vi "Demo Main BSC.vi"() -> ()   [LabVIEW 2022 SP3]
uses:
  Logo.ctl
  C:/Users/Public/OneDrive/Desktop/PMT program/SampleCodeLabView/Kinesis_with_LabVIEW_Examples_LV12 - v3/Thorlabs.MotionControl.Controls.dll
  Kinesis_with_LabVIEW_Examples_LV12 - v3/Thorlabs.MotionControl.Controls.dll
  C:/Users/Public/OneDrive/Desktop/PMT program/SampleCodeLabView/Kinesis_with_LabVIEW_Examples_LV12 - v3/Thorlabs.MotionControl.Benchtop.StepperMotorCLI.dll
  Kinesis_with_LabVIEW_Examples_LV12 - v3/Thorlabs.MotionControl.Benchtop.StepperMotorCLI.dll
  <vilib>/Utility/file.llb/Write Delimited Spreadsheet (string).vi
  <vilib>/Utility/file.llb/Write Delimited Spreadsheet (I64).vi
  <vilib>/Utility/file.llb/Write Delimited Spreadsheet (DBL).vi
  C:/Users/Public/OneDrive/Desktop/PMT program/SampleCodeLabView/Kinesis_with_LabVIEW_Examples_LV12 - v3/Thorlabs.MotionControl.GenericMotorCLI.dll
  Kinesis_with_LabVIEW_Examples_LV12 - v3/Thorlabs.MotionControl.GenericMotorCLI.dll
  <vilib>/Analysis/NI_AALBase.lvlib
panel:
  out "ESD":i32=1 caption="Steps\nAdded/Removed"
  in  "ES":i32=1 caption="Add /Remove \nSteps" format="%.0g"
  out "Sweep Graph":u32[](graph)=[692, 692, 717, 859, 1299, 1810, 1150, 733, 722, 683, 685, 676, 665, 671, 1299, 1362, 1395, 1437, 1460, 1539, 1625, 1626, 1658, 1682, 1737, 1780, 1784, 1780, 1793, 1801, 1778, 1738, 1746, 1700, 1643, 1578, 1545, 1504, 1448, 1394, 1310, 1272, 1209, 1133, 1067, 1028, 991, 955, 889, 855, 832, 810, 790, 767, 743, 738, 724, 715, 709, 699, 697, 691, 696, 694, 695, 710, 710, 694, 696, 690, 687, 684, 682, 689, 668]
  out "SM":i32 caption="Sweep\nMean"
  out "SN":i32=61 caption="Current Sweep Iteration"
  out "SND":i32=61 caption="Total No. of Sweeps"
  in  "Auto-Sweep":bool
  in  "P8":bool
  out "PC":dbl=1810482.0 caption="Current \nPosition" format="%#_6f"
  out "WTD":i32=2000 caption="Wait Time (ms)\nRead Data"
  out "EPD":dbl=70.72 caption="End Position\nRead Data"
  out "SPD":dbl=70.66 caption="Start Position\nRead Data"
  out "SSD":dbl=0.001 caption="Step Size\nRead Data" format="%.4g"
  in  "SP":dbl=70.66 caption="Start Position (degrees)\n Set Data"
  in  "WT":i32=2000 caption="Wait Time (ms)\n Set Data"
  in  "EP":dbl=70.72 caption="End Position (degrees)\n Set Data"
  in  "P7":bool
  in  "SS":dbl=0.001 caption="Step Size (degrees)\nSet Data"
  in  "Motor Controller\nSerialNumber":string="40837323"
  in  "BenchtopStepperControl":refnum<k24>(container)
  in  "Export":bool
  out "DB":u32[](array[numeric])=[729, 0, 0, 0, 0, 0, 0, 0, 0, 0, 0, 0, 0, 0, 0, 0]
  out "OVL":bool caption="LED ON : Over Rang Data"
  out "OLD":i32
  out "GN":i32 caption="Gate Number"
  in  "Correction":bool=TRUE
  in  "Logo":T1
  out "Graph":u32[](graph)=[729]
  in  "Stop":bool
  in  "Start":bool
  in  "P6":bool
  out "RND":i32=40 caption="Read Number\nRead Data"
  in  "P5":bool
  in  "RN":i32=40 caption="Read Number\nSet Data"
  out "PowerD":i32=1 caption="Power\nRead Data"
  out "ITD":i32=100 caption="Internal Time\nRead Data"
  in  "P4":bool
  in  "P3":bool
  in  "IT":i32=100 caption="Internal Time\nSet Data"
  in  "P2":bool
  out "Handle Number":i32=169470376
  in  "P1":bool caption="Switch\nPower OFF/Power ON"
  in  "EXIT":bool=TRUE
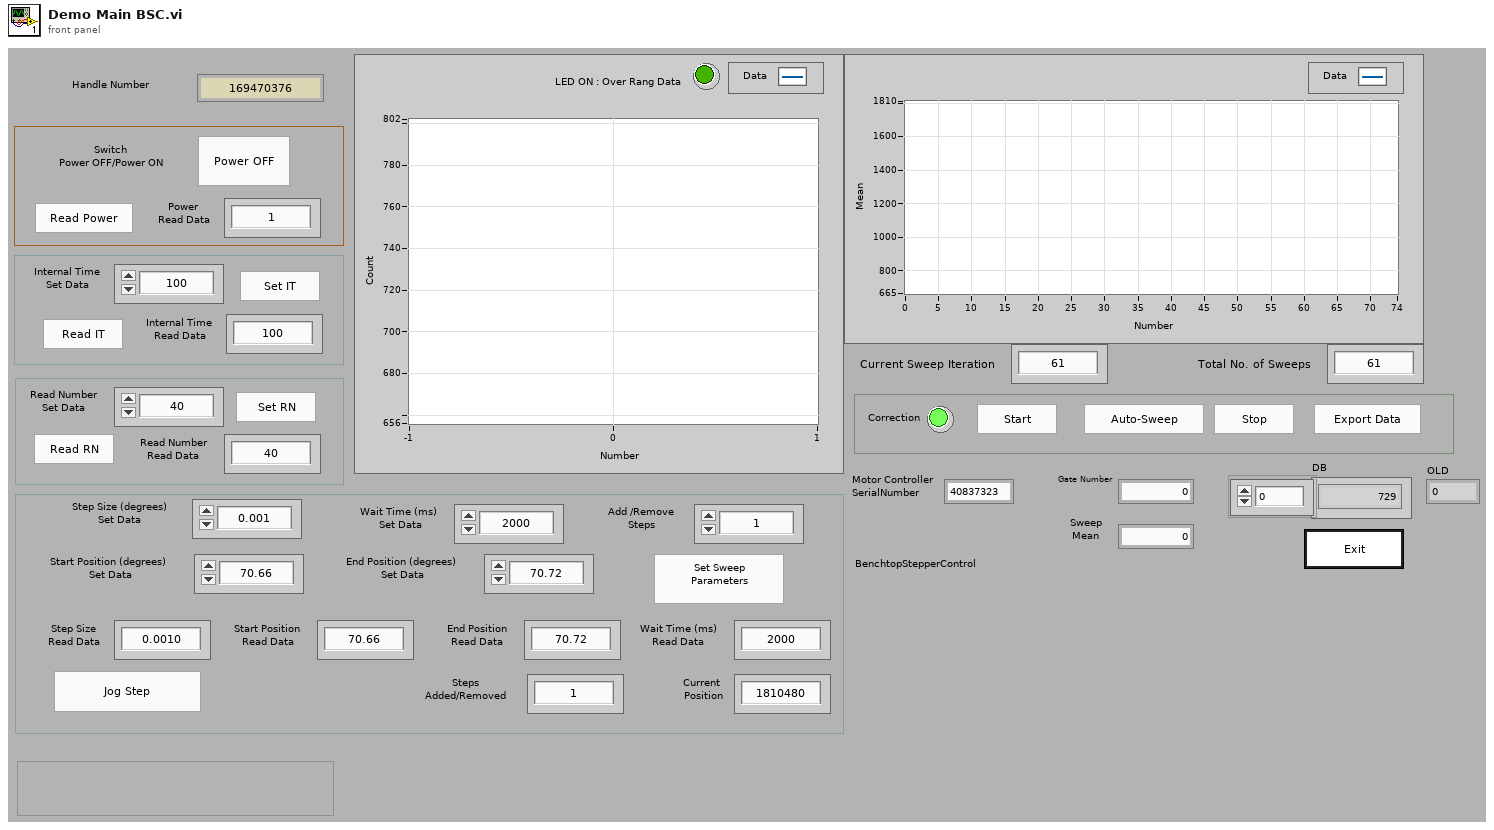
[diagram p1: front panel]
types:
  T1 = typedef "Logo.ctl" = bool
  T2 = enum8{"Enabled", "Disabled", "Disabled and Grayed Out"}
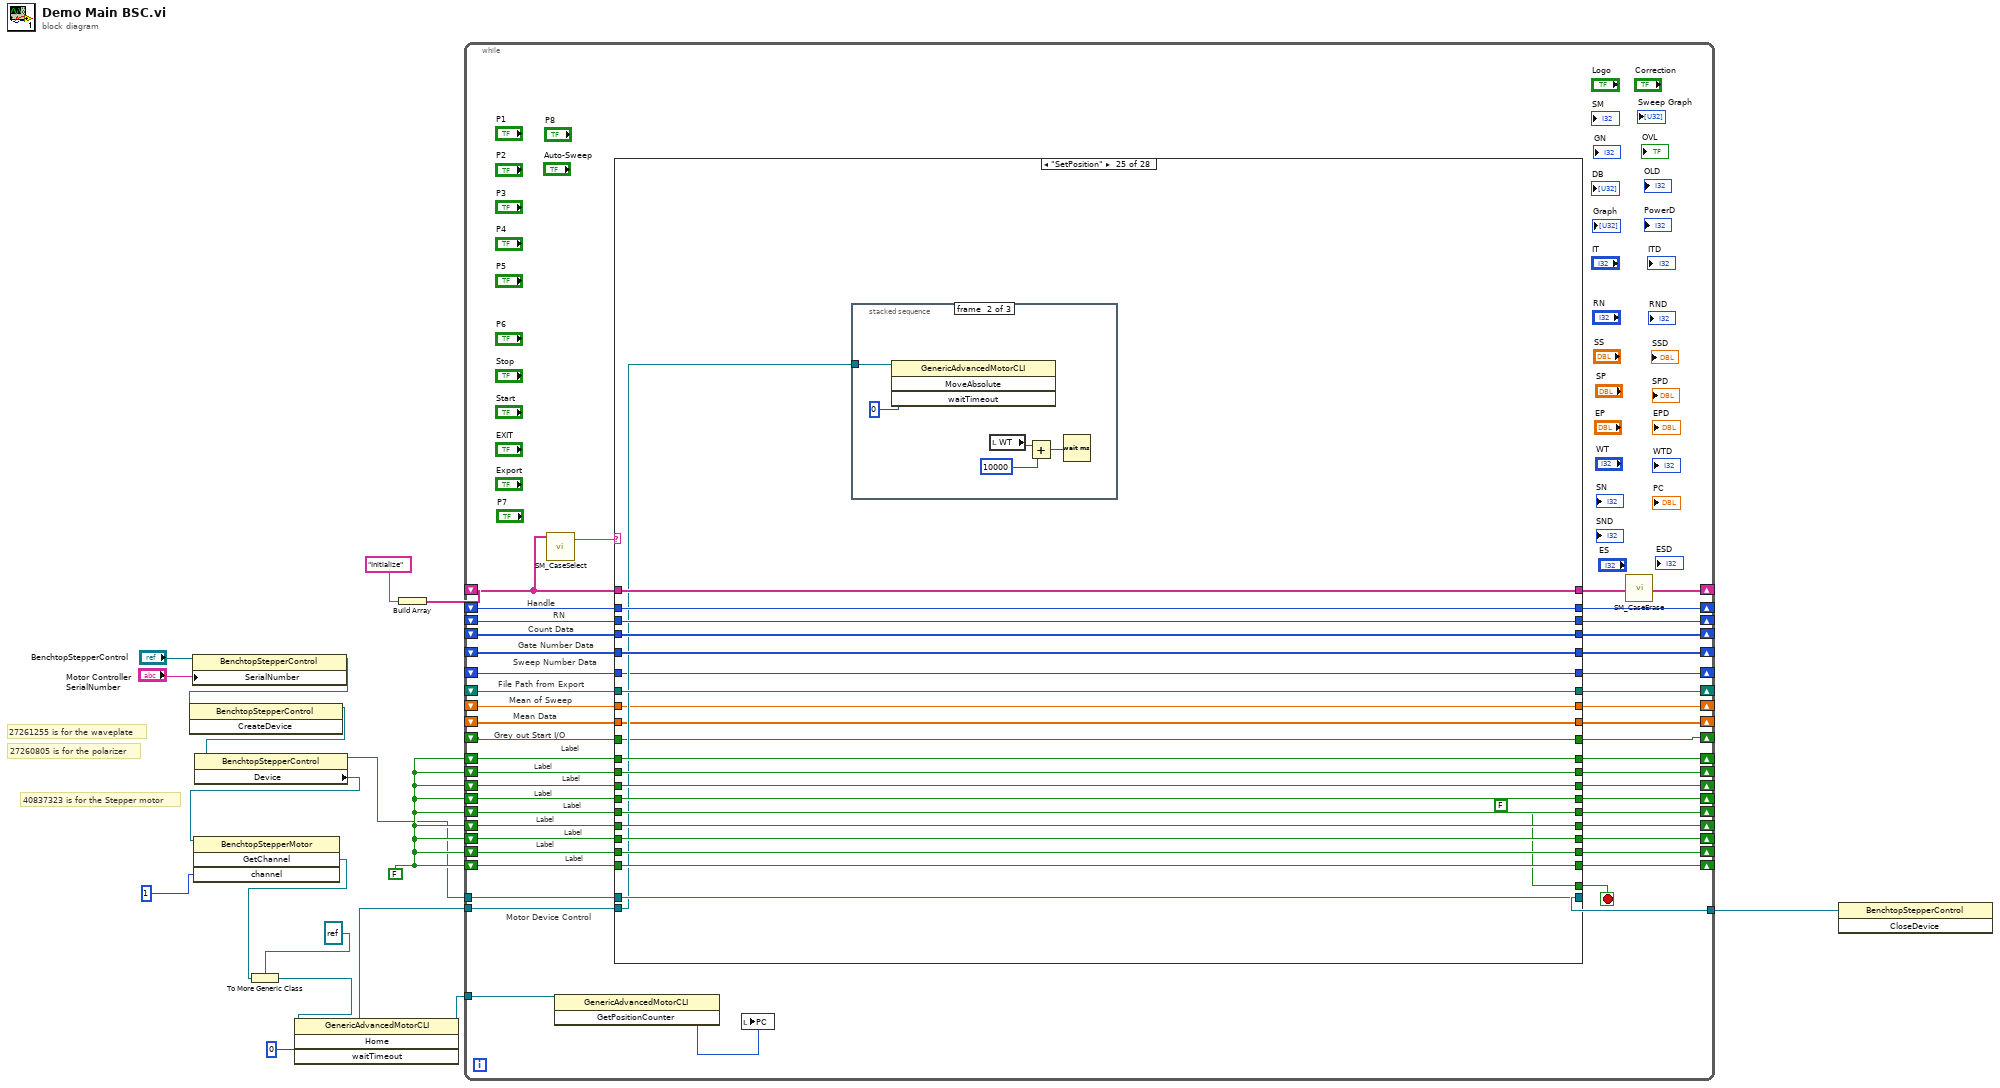
[diagram p0: block diagram]
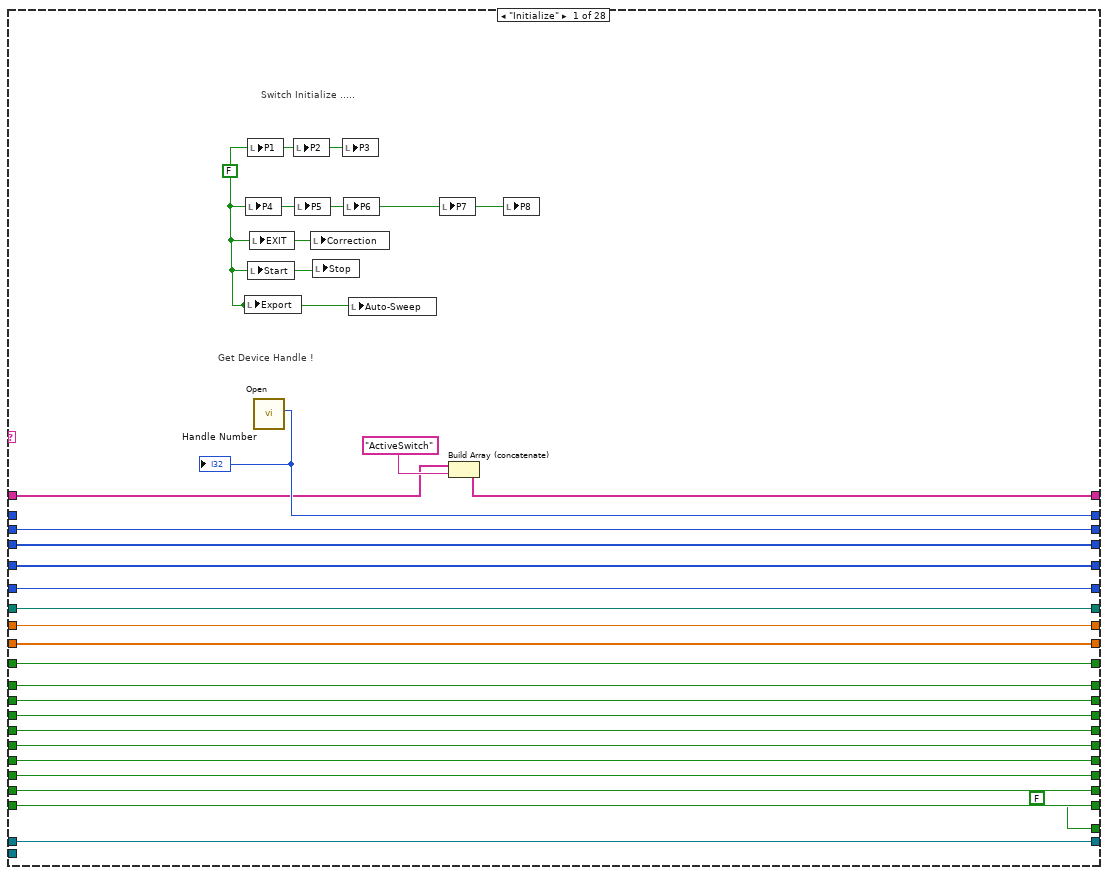
[diagram p2: hidden frame]
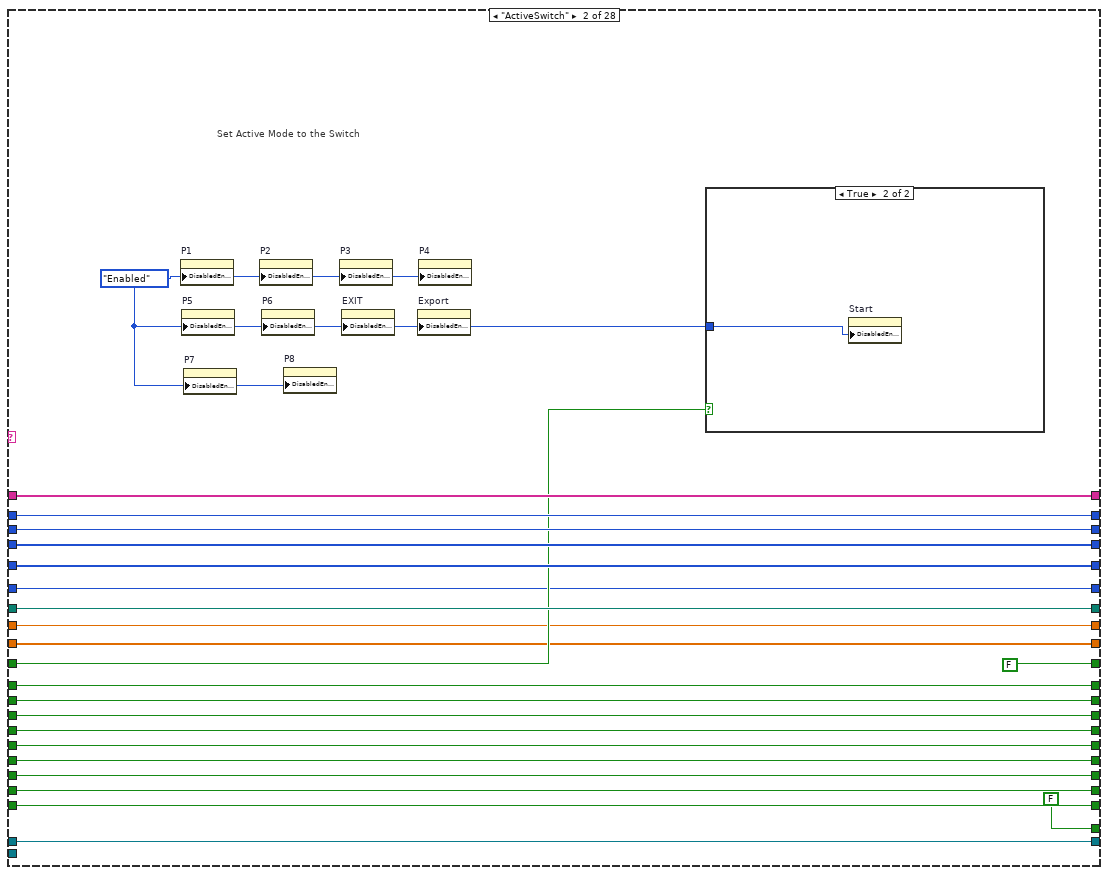
[diagram p3: hidden frame]
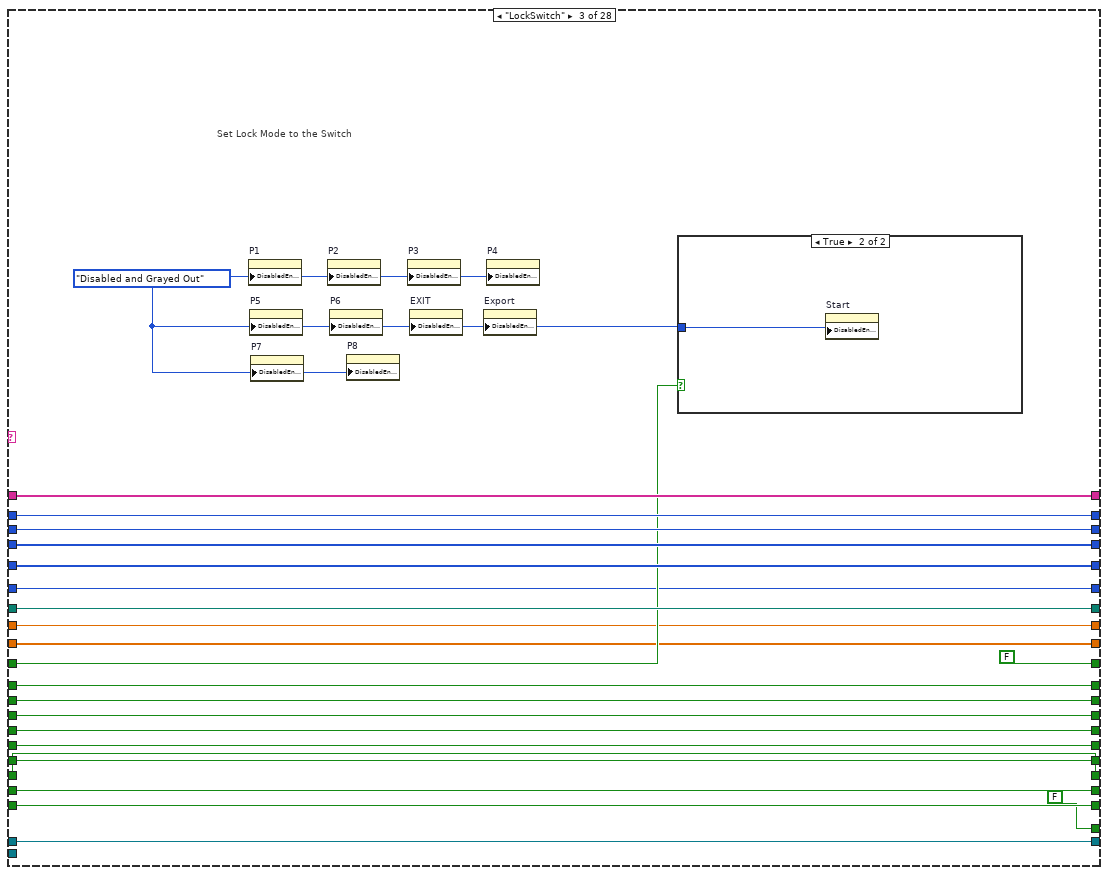
[diagram p5: hidden frame]
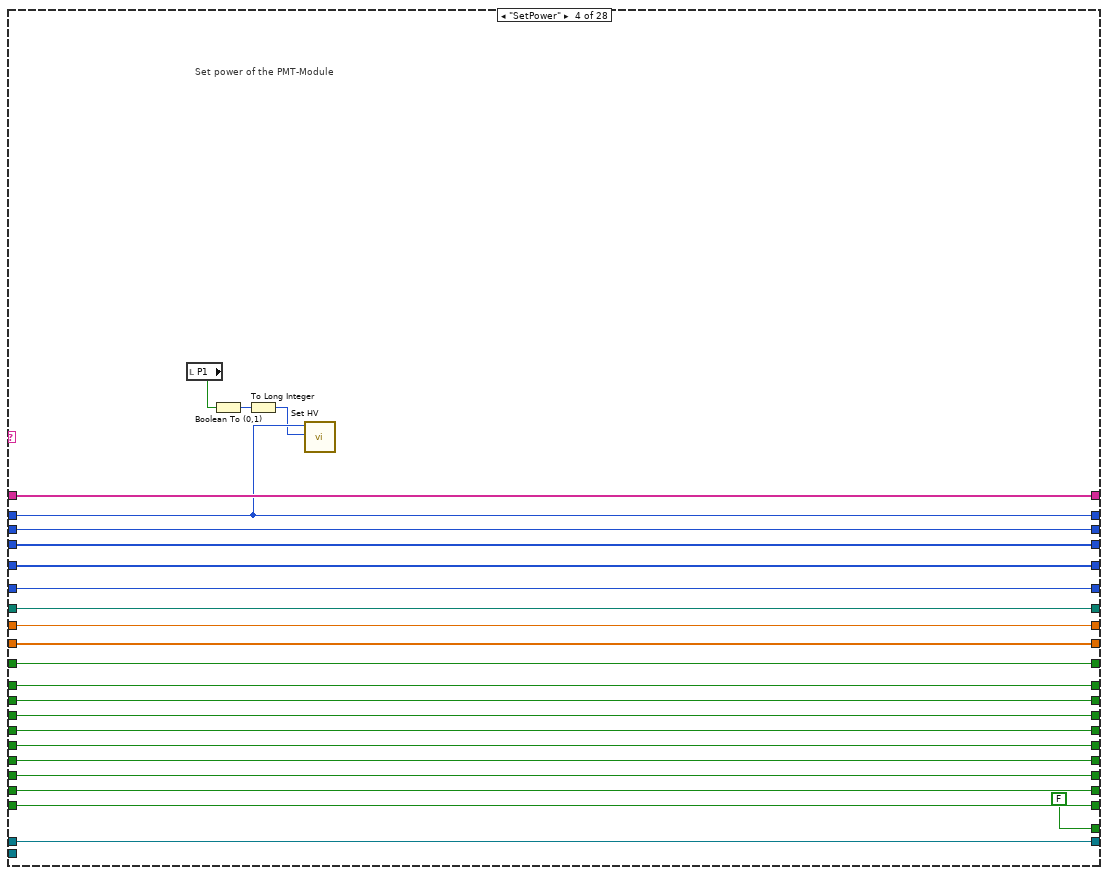
[diagram p7: hidden frame]
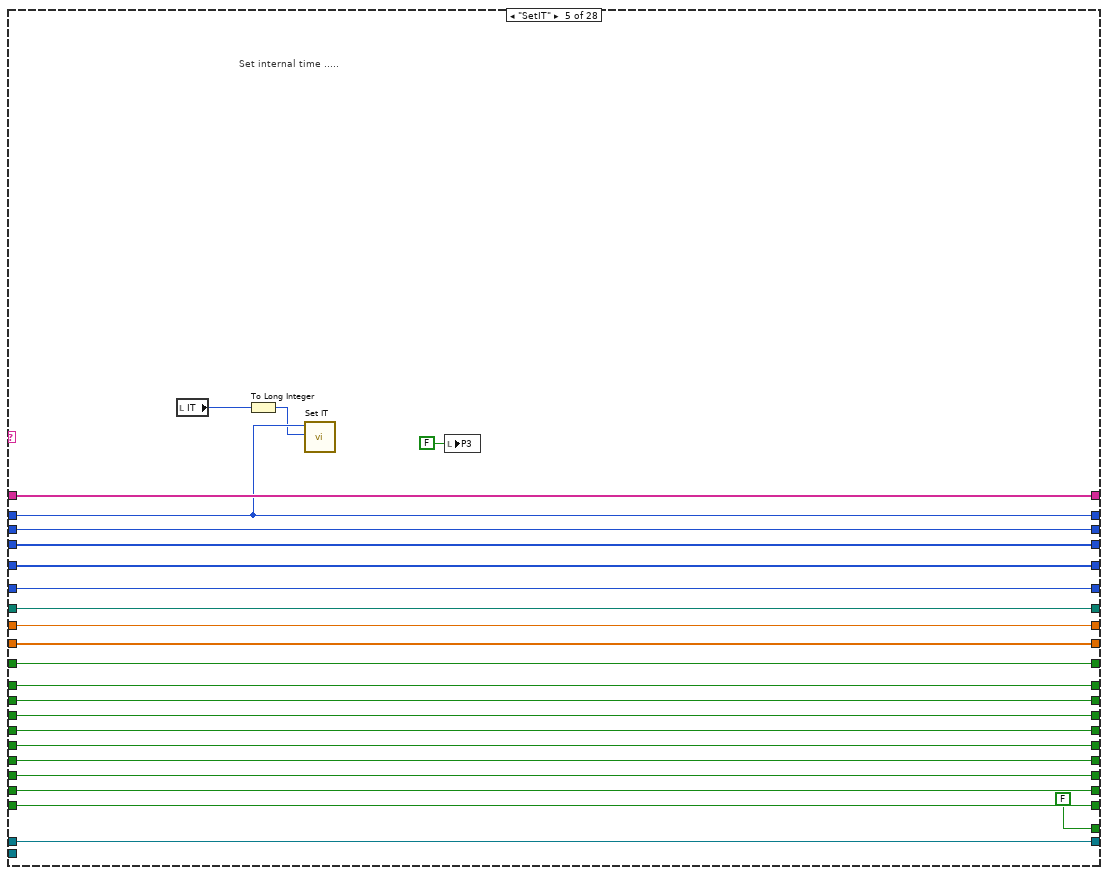
[diagram p8: hidden frame]
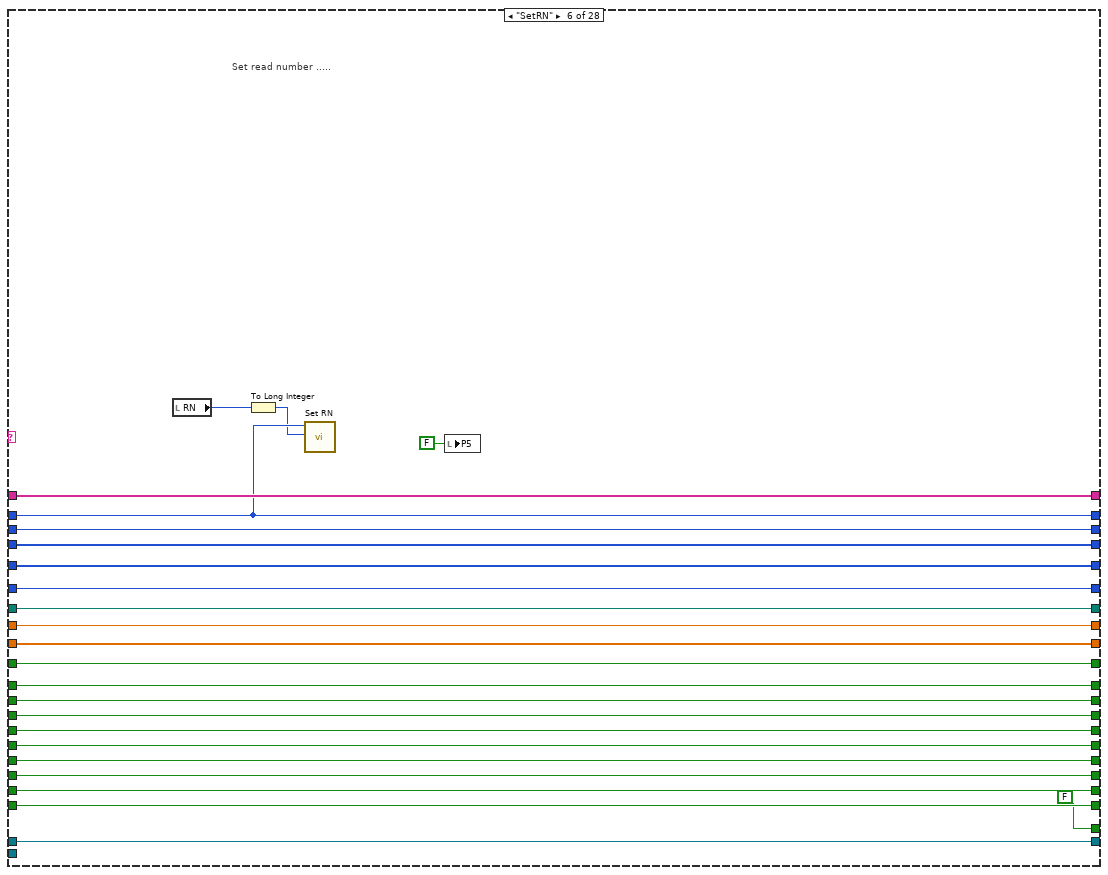
[diagram p9: hidden frame]
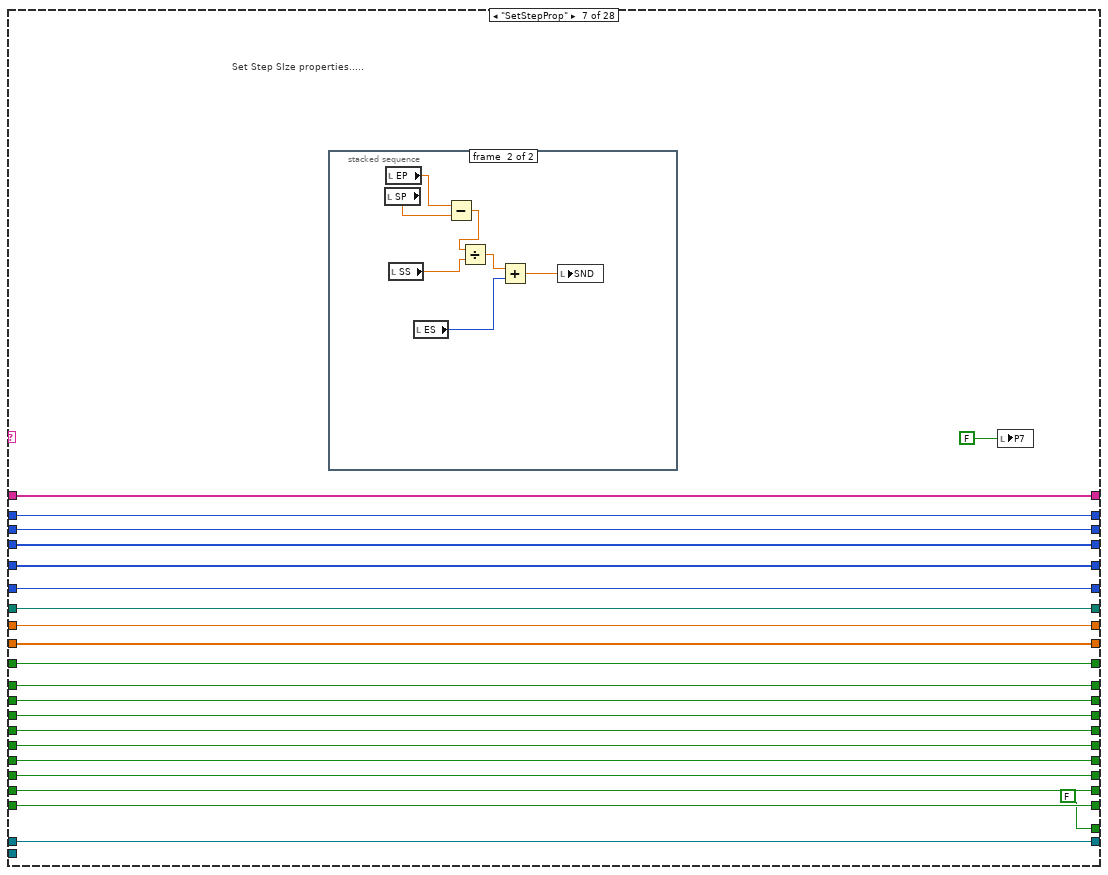
[diagram p10: hidden frame]
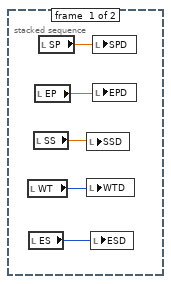
[diagram p11: hidden frame]
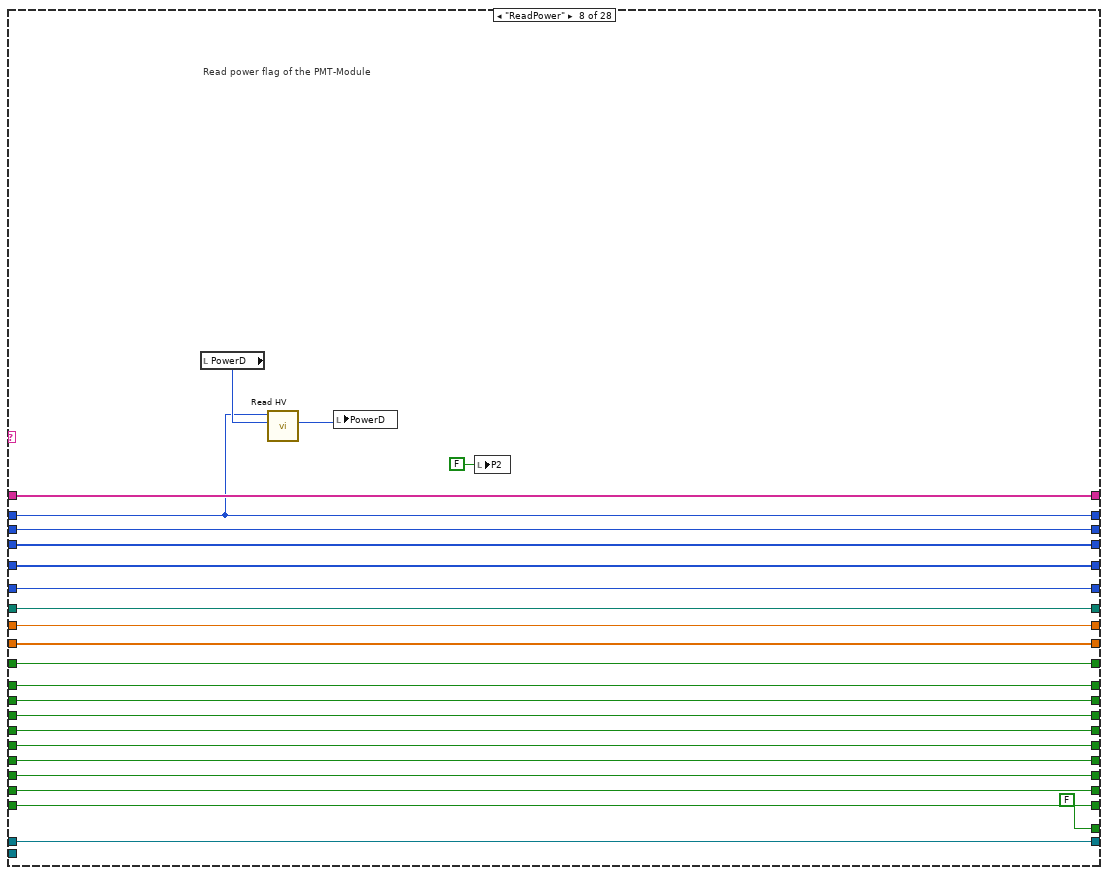
[diagram p12: hidden frame]
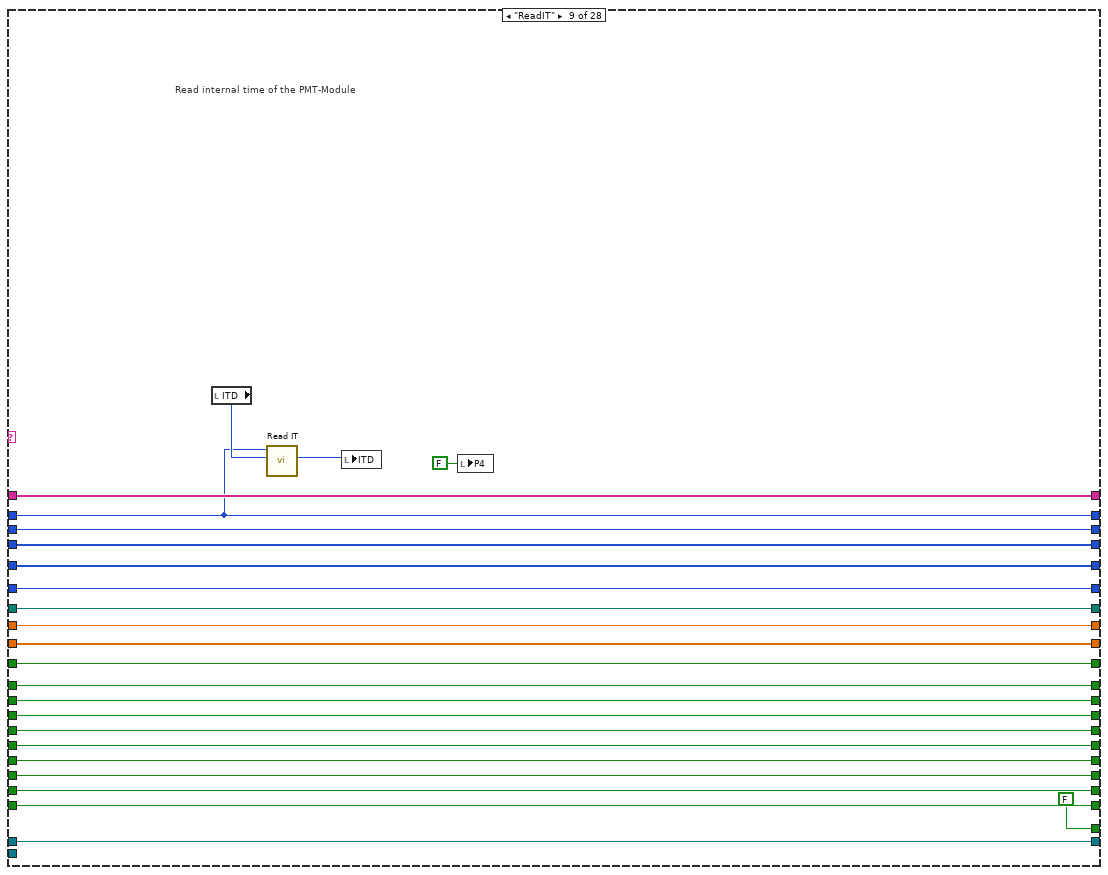
[diagram p13: hidden frame]
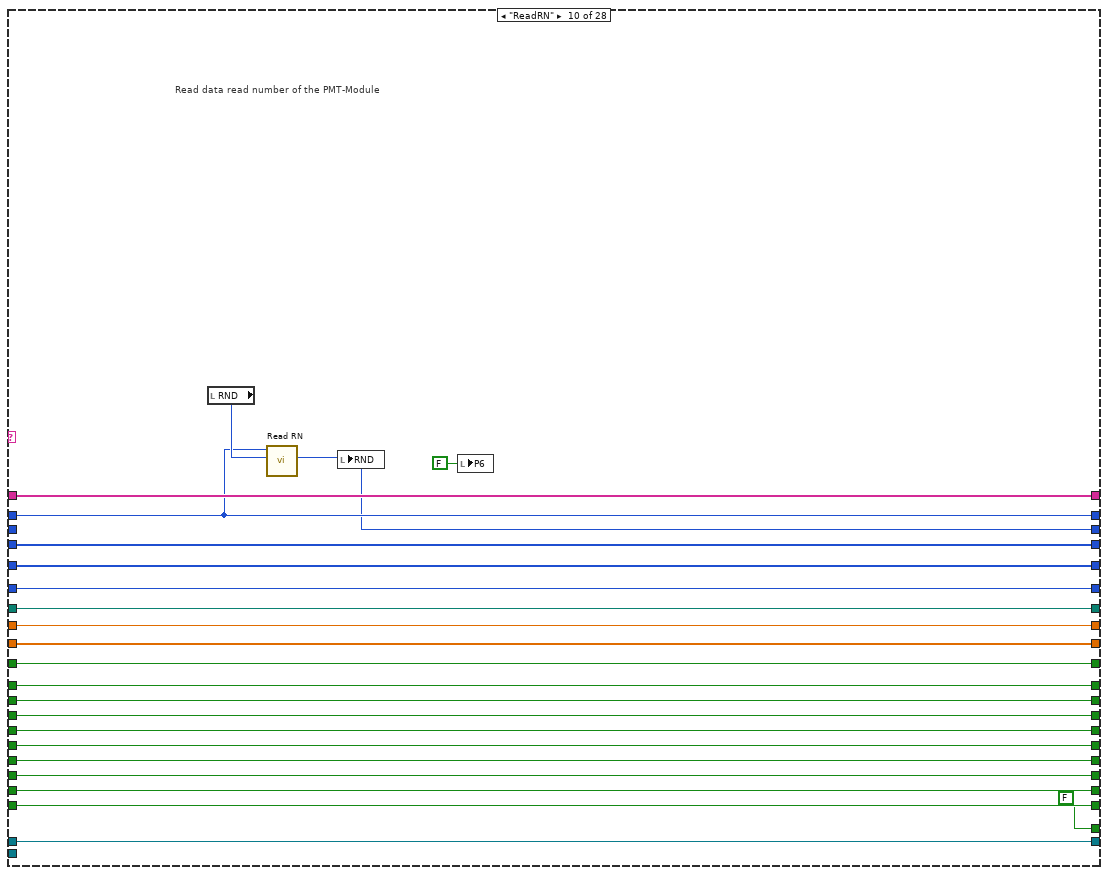
[diagram p14: hidden frame]
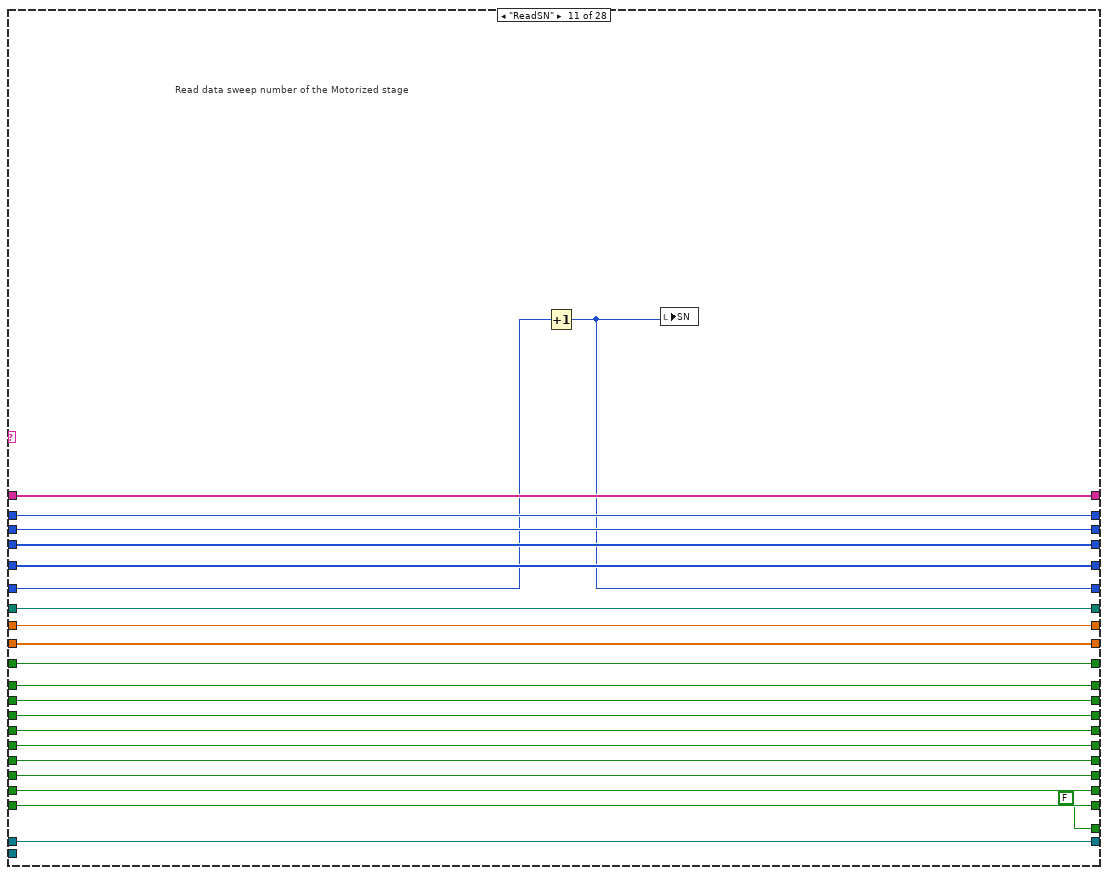
[diagram p15: hidden frame]
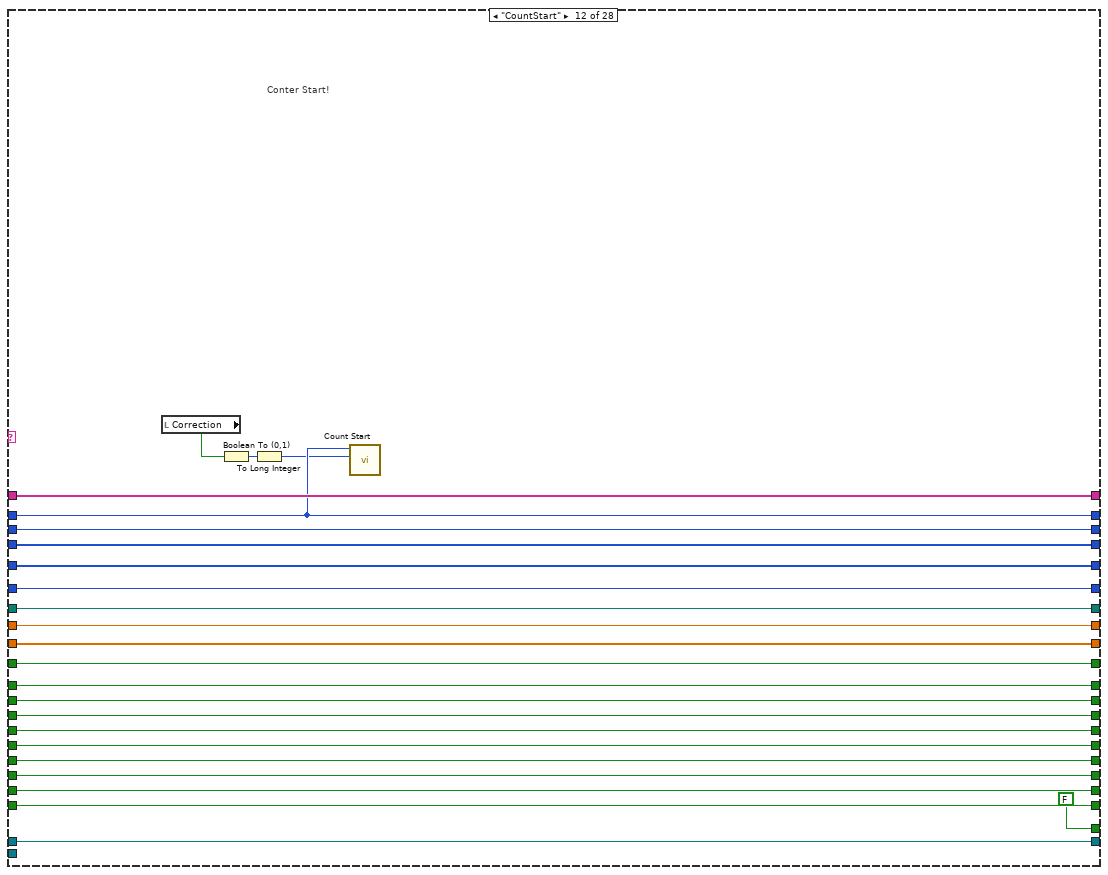
[diagram p16: hidden frame]
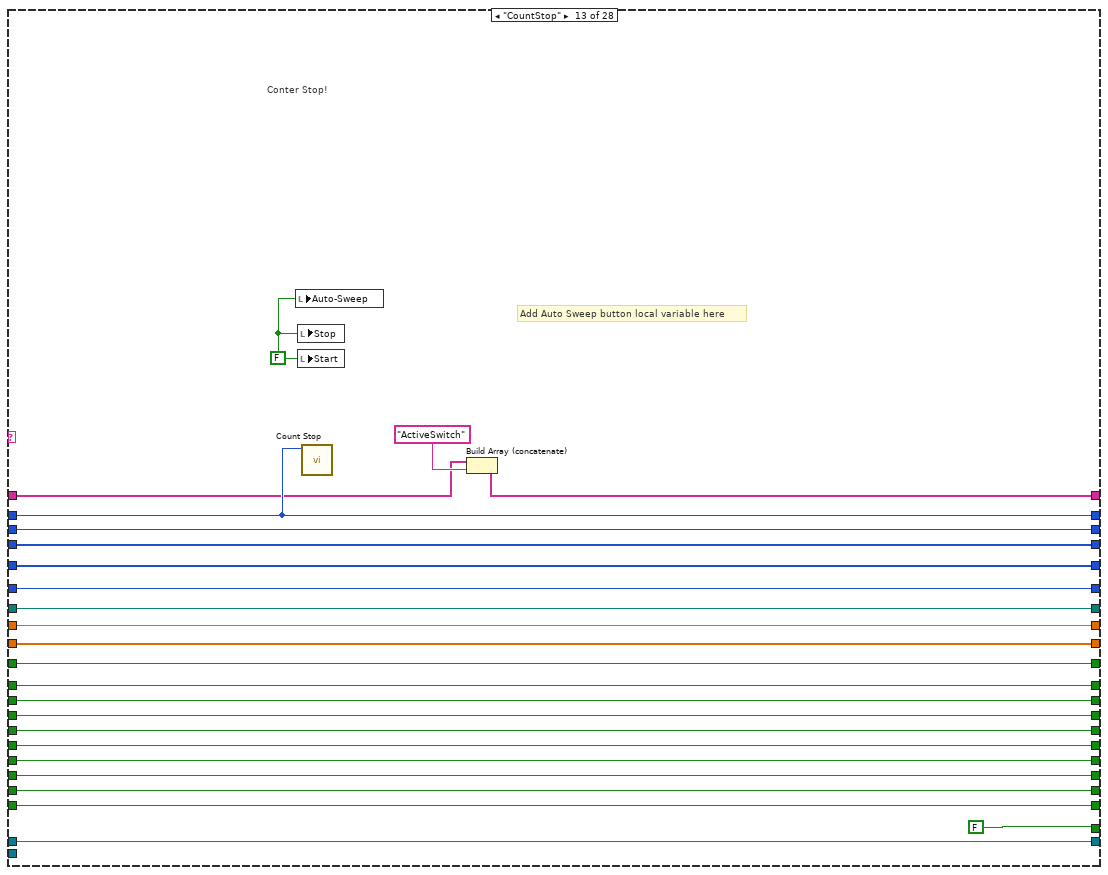
[diagram p17: hidden frame]
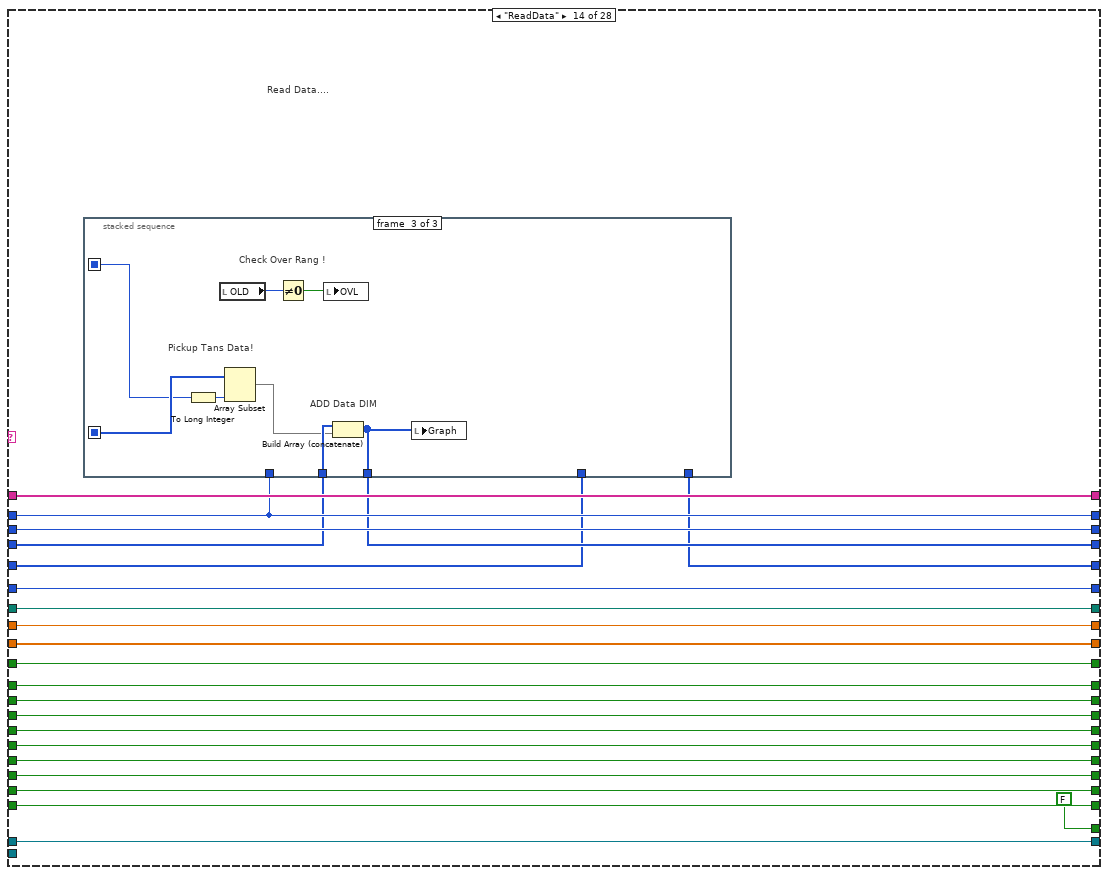
[diagram p18: hidden frame]
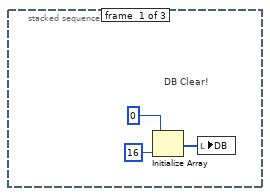
[diagram p19: hidden frame]
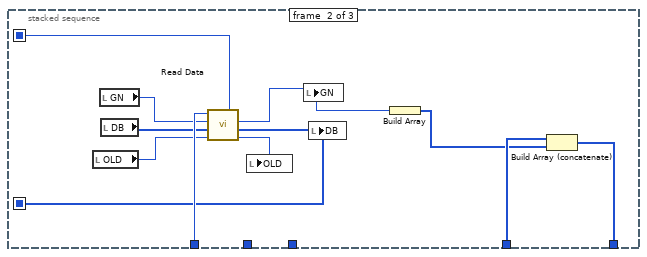
[diagram p20: hidden frame]
diagram:
  w14 = FALSE
  # "40837323 is for the Stepper motor"
  # "27260805 is for the polarizer"
  # "27261255 is for the waveplate"
  n1 = property class="BenchtopStepperControl"(reference="BenchtopStepperControl", "SerialNumber"="Motor Controller\nSerialNumber") -> (reference out=w12:refnum<k24>)  [unwired: 1 in, 1 out]
  n2 = invoke class="BenchtopStepperControl" method="CreateDevice"(reference=w12) -> (reference out=w6:refnum<k24>)  [unwired: 2 in, 2 out]
  n3 = property class="BenchtopStepperControl"(reference=w6) -> (reference out=w9:refnum<k24>, "Device"=w4:refnum<k24>)  [unwired: 1 in, 1 out]
  n4 = invoke class="BenchtopStepperMotor" method="GetChannel"(reference=w4, "channel"=1) -> ("GetChannel"=w3:refnum<k24>)  [unwired: 2 in, 3 out]
  n5 = To More Generic Class(target class=refnum<k24> refnum, reference=w3) -> (generic class reference=w1:refnum<k24>)
  n6 = invoke class="GenericAdvancedMotorCLI" method="Home"(reference=w1, "waitTimeout"=0) -> (reference out=w7:refnum<k24>)  [unwired: 2 in, 3 out]
  n7 = Build Array("Initialize") -> (w15:string[])
  n8 = while {
    shift-right: [w45] -> _
    shift-left: w14 -> [w46]
    shift-right: [w47] -> _
    shift-left: w14 -> [w48]
    shift-right: [w49] -> _
    shift-left: w14 -> [w50]
    shift-right: [w51] -> _
    shift-left: w14 -> [w52]
    shift-right: [w53] -> _
    shift-left: _ -> [w54]
    shift-right: [w55] -> _
    shift-left: _ -> [w56]
    shift-right: [w57] -> _
    shift-left: _ -> [w58]
    shift-right: [w43] -> _
    shift-left: w14 -> [w44]
    shift-right: [w61] -> _
    shift-left: w14 -> [w62]
    shift-right: [w40] -> _
    shift-left: w15 -> [w59]
    shift-right: [w38] -> _
    shift-left: w14 -> [w39]
    shift-right: [w36] -> _
    shift-left: w14 -> [w37]
    shift-right: [w35] -> _
    shift-left: w14 -> [w34]
    tunnel: w9 -> [w31]
    tunnel: [w30] -> w10
    shift-right: [w33] -> _
    shift-left: _ -> [w32]
    tunnel: w1 -> [w29]
    shift-right: [w28] -> _
    shift-left: _ -> [w27]
    shift-right: [w26] -> _
    shift-left: _ -> [w25]
    tunnel: w7 -> [w24]
    shift-right: [w22] -> _
    shift-left: _ -> [w23]
    shift-right: [w21] -> _
    shift-left: _ -> [w20]
    shift-right: [w19] -> _
    shift-left: _ -> [w18]
    stop <- w42 stop-if-true
    # "Mean Data"
    # "Mean of Sweep"
    # "Sweep Number Data"
    # "Grey out Start I/O"
    # "Motor Device Control"
    # "File Path from Export"
    # "Gate Number Data"
    # "Label"
    # "Label"
    # "Label"
    # "Label"
    # "Label"
    # "Label"
    # "Label"
    # "Label"
    # "Label"
    # "Count Data"
    # "RN"
    # "Handle"
    n9 = call "SM_CaseSelect.vi"("Input"=w59) -> ("Case"=w60:string)  [unwired: 10 out]
    n10 = invoke class="GenericAdvancedMotorCLI" method="GetPositionCounter"(reference=w24) -> ("GetPositionCounter"=w17:i32)  [unwired: 2 in, 2 out]
    n11 = case shown="\"SetPosition\"" w60 {
      selector: w60 -> [_ _ _ _ _ _ _ _ _ _ _ _ _ _ _ _ _ _ _ _ _ _ _ _ _ _ w938 _]
      tunnel: w62 -> [w86 w109 w133 w158 w182 w206 w228 w264 w288 w311 w333 w357 w381 w404 w448 w479 w505 w545 w583 w652 w705 w756 w786 w808 w838 w885 w956 w977]
      tunnel: [w86 w109 w133 w158 w182 w206 w228 w264 w288 w311 w333 w357 w381 w404 w448 w479 w505 w545 w583 w652 w705 w756 w786 w808 w838 w885 w956 w977] -> w61
      tunnel: w59 -> [w72 w108 w132 w157 w181 w205 w227 w263 w287 w310 w332 w356 w367 w403 w447 w467 w483 w532 w571 w663 w716 w767 w778 w821 w851 w873 w955 w976]
      tunnel: [w71 w108 w132 w157 w181 w205 w227 w263 w287 w310 w332 w356 w366 w403 w447 w466 w482 w533 w572 w663 w716 w767 w777 w821 w851 w870 w955 w976] -> w41
      tunnel: w58 -> [_ w96 w120 w145 w169 w193 w215 w250 w274 w298 w321 w344 w369 w392 w436 w468 w494 w535 w573 w662 w715 w766 w798 w820 w850 w884 w954 w964]
      tunnel: [w74 w96 w120 w145 w169 w193 w215 w250 w274 w298 w321 w344 w369 w392 w436 w468 w494 w535 w573 w662 w715 w766 w798 w820 w850 w884 w954 w964] -> w57
      tunnel: w56 -> [w85 w107 w131 w156 w180 w204 w226 w262 w286 _ w314 w355 w380 w402 w446 w478 w504 w530 w569 w661 w714 w765 w797 w819 w849 w883 w953 w975]
      tunnel: [w85 w107 w131 w156 w180 w204 w226 w262 w286 w296 w314 w355 w380 w402 w446 w478 w504 w530 w569 w661 w714 w765 w797 w819 w849 w883 w953 w975] -> w55
      tunnel: w54 -> [w84 w106 w130 w155 w179 w203 w225 w261 w285 w309 w331 w354 w379 w391 w431 _ _ w526 w567 w637 w690 w741 w796 w818 w848 w869 w952 w974]
      tunnel: [w84 w106 w130 w155 w179 w203 w225 w261 w285 w309 w331 w354 w379 w390 w431 w458 w492 w526 w567 w637 w690 w741 w796 w818 w848 w869 w952 w974] -> w53
      tunnel: w52 -> [w83 w105 w129 w154 w178 w202 w224 w260 w284 w308 w330 w353 w378 w401 w445 w477 w503 w544 w582 w660 w713 w764 w794 w816 w846 w882 w951 w973]
      tunnel: [w83 w105 w129 w154 w178 w202 w224 w260 w284 w308 w330 w353 w378 w401 w445 w477 w503 w544 w582 w660 w713 w764 w794 w816 w846 w882 w951 w973] -> w51
      tunnel: w50 -> [w82 w104 w128 w153 w177 w201 w223 w259 w283 w307 w329 w352 w377 w400 w444 w476 w502 w543 w581 w659 w712 w763 w793 w815 w845 w881 w950 w972]
      tunnel: [w82 w104 w128 w153 w177 w201 w223 w259 w283 w307 w329 w352 w377 w400 w444 w476 w502 w543 w581 w659 w712 w763 w793 w815 w845 w881 w950 w972] -> w49
      tunnel: w48 -> [w81 w103 w127 w152 w176 w200 w222 w258 w282 w306 w328 w351 w376 w399 w443 w475 w501 w542 w580 w658 w711 w762 w792 w814 w844 w880 w949 w971]
      tunnel: [w81 w103 w127 w152 w176 w200 w222 w258 w282 w306 w328 w351 w376 w399 w443 w475 w501 w542 w580 w658 w711 w762 w792 w814 w844 w880 w949 w971] -> w47
      tunnel: w46 -> [w80 w102 w126 w151 w175 w199 w221 w257 w281 w305 w327 w350 w375 w398 w442 w474 w500 w541 w579 w657 w710 w761 w791 w813 w843 w879 w948 w970]
      tunnel: [w80 w102 w126 w151 w175 w199 w221 w257 w281 w305 w327 w350 w375 w398 w442 w474 w500 w541 w579 w657 w710 w761 w791 w813 w843 w879 w948 w970] -> w45
      tunnel: w44 -> [w79 w101 w125 w150 w174 w198 w220 w256 w280 w304 w326 w349 w374 w397 w441 w473 w499 w540 w578 w656 w709 w760 w790 w812 w842 w878 w947 w969]
      tunnel: [w79 w101 w125 w150 w174 w198 w220 w256 w280 w304 w326 w349 w374 w397 w441 w473 w499 w540 w578 w656 w709 w760 w790 w812 w842 w878 w947 w969] -> w43
      tunnel: [FALSE FALSE FALSE FALSE FALSE FALSE FALSE FALSE FALSE FALSE FALSE FALSE FALSE FALSE FALSE FALSE FALSE FALSE FALSE FALSE FALSE FALSE FALSE FALSE FALSE FALSE FALSE TRUE] -> w42
      tunnel: w39 -> [w75 w97 w121 w146 w170 w194 w216 w252 w276 w300 w322 w345 w370 w393 w437 w469 w495 w536 w574 w655 w708 w759 w789 w811 w841 w874 w943 w965]
      tunnel: [w75 w97 w121 w146 w170 w194 w216 w252 w276 w300 w322 w345 w370 w393 w437 w469 w495 w536 w574 w655 w708 w759 w789 w811 w841 w874 w943 w965] -> w38
      tunnel: w37 -> [w77 w99 w123 w148 w172 w196 w218 w254 w278 w302 w324 w347 w372 w395 w439 w471 w497 w538 w576 w654 w707 w758 w788 w810 w840 w876 w945 w967]
      tunnel: [w77 w99 w123 w148 w172 w196 w218 w254 w278 w302 w324 w347 w372 w395 w439 w471 w497 w538 w576 w654 w707 w758 w788 w810 w840 w876 w945 w967] -> w36
      tunnel: [w76 w98 w122 w147 w171 w195 w217 w253 w277 w301 w323 w346 w371 w394 w438 w470 w496 w537 w575 w653 w706 w757 w787 w809 w839 w875 w944 w966] -> w35
      tunnel: w34 -> [w76 w98 w122 w147 w171 w195 w217 w253 w277 w301 w323 w346 w371 w394 w438 w470 w496 w537 w575 w653 w706 w757 w787 w809 w839 w875 w944 w966]
      tunnel: [w70 w95 w119 w141 w165 w189 w214 w247 w271 w295 w320 w340 w365 w389 w430 w458 w492 w525 w566 w632 w685 w736 w795 w817 w847 w868 w937 w963] -> w33
      tunnel: w32 -> [w70 w95 w119 w141 w165 w189 w214 w247 w271 w295 w320 w340 w365 w388 w430 _ _ w525 w566 w632 w685 w736 w795 w817 w847 w868 w937 w963]
      tunnel: w31 -> [w69 w94 w118 w140 w164 w188 w213 w246 w270 w294 w319 w339 w364 w387 w435 w457 w491 w524 w565 w634 w687 w738 w785 w807 w837 w867 w936 w962]
      tunnel: [w69 w94 w118 w140 w164 w188 w213 w246 w270 w294 w319 w339 w364 w387 w435 w457 w491 w524 w565 w634 w687 w738 w785 w807 w837 w867 w936 w962] -> w30
      tunnel: w29 -> [_ _ _ _ _ _ _ _ _ _ _ _ _ _ _ _ _ _ _ _ _ _ _ w804 w834 _ _ _]
      tunnel: [w68 w93 w117 w139 w163 w187 w211 w245 w269 w293 w318 w338 w363 w386 w434 w456 w490 w523 w564 w625 w681 w732 w774 w805 w835 w866 w935 w961] -> w28
      tunnel: w27 -> [w68 w93 w117 w139 w163 w187 w211 w245 w269 w293 w318 w338 w363 w386 w434 w456 w490 w523 w564 w625 w677 w730 _ w805 w835 w866 w935 w961]
      tunnel: [w67 FALSE FALSE w138 w162 w186 w210 w244 w268 w292 w317 w337 w362 w385 w433 w455 TRUE w522 w563 w627 w680 w731 w783 w803 w833 w865 w934 w960] -> w26
      tunnel: w25 -> [w67 w92 w116 w138 w162 w186 w210 w244 w268 w292 w317 w337 w362 w385 w433 w455 _ w522 _ w627 w680 w731 w783 w803 w833 w865 w934 w960]
      tunnel: w23 -> [w65 w89 w113 w137 w161 w185 w209 w243 w267 w291 w312 w336 w361 w384 w432 w454 w488 w521 w562 w626 w673 w727 _ w799 w832 w864 w933 w959]
      tunnel: [w65 w89 w113 w137 w161 w185 w209 w243 w267 w291 w313 w336 w361 w384 w432 w454 w488 w521 w562 w626 w673 w727 w775 w799 w832 w864 w933 w959] -> w22
      tunnel: [w64 w88 w112 w136 w160 w184 w208 w242 w266 w290 w316 w335 w360 w383 w429 w453 w487 w520 w559 w624 w679 w729 w782 w801 w831 w863 w932 w958] -> w21
      tunnel: w20 -> [w64 w88 w112 w136 w160 w184 w208 w242 w266 w290 w316 w335 w360 w383 w429 w453 w487 w520 w559 w624 _ _ w782 w801 w831 w863 w932 w958]
      tunnel: [w63 w87 w111 w135 w159 w183 w207 w241 w265 w289 w315 w334 w359 w382 w428 w452 w486 w519 w558 w623 w678 w728 w776 w800 w830 w862 w931 w957] -> w19
      tunnel: w18 -> [w63 w87 w111 w135 w159 w183 w207 w241 w265 w289 w315 w334 w359 w382 w427 w452 w486 w519 w558 w623 w678 w728 w776 w800 w830 w862 w931 w957]
      frame "Initialize" {
        w66 = FALSE ("P1")
        # "Get Device Handle !"
        # "Switch Initialize ....."
        n12 = local write "Export"(w66) -> ()
        n13 = local write "P4"(w66) -> ()
        n14 = local write "P1"(w66) -> ()
        n15 = local write "Start"(w66) -> ()
        n16 = local write "EXIT"(w66) -> ()
        n17 = call "Open.vi"() -> ("Handle Number"=w74:i32)  [unwired: 10 in, 1 out]
        "Handle Number" <- w74
        n18 = local write "P2"(w66) -> ()
        n19 = local write "P5"(w66) -> ()
        n20 = local write "Correction"(w66) -> ()
        n21 = local write "Stop"(w66) -> ()
        n22 = local write "P3"(w66) -> ()
        n23 = local write "P6"(w66) -> ()
        n24 = local write "Auto-Sweep"(w66) -> ()
        n25 = local write "P7"(w66) -> ()
        n26 = Build Array (concatenate)(w72, "ActiveSwitch") -> (w71:string[])
        n27 = local write "P8"(w66) -> ()
      }
      frame "ActiveSwitch" {
        w90 = T2."Enabled" ("無効")
        # "Set Active Mode to the Switch"
        n28 = property on="P1" class="Bool (strict)"("DisabledEnum"=w90) -> ()  [unwired: 2 in, 2 out]
        n29 = property on="P5" class="Bool (strict)"("DisabledEnum"=w90) -> ()  [unwired: 2 in, 2 out]
        n30 = property on="P7" class="Bool (strict)"("DisabledEnum"=w90) -> ()  [unwired: 2 in, 2 out]
        n31 = property on="P2" class="Bool (strict)"("DisabledEnum"=w90) -> ()  [unwired: 2 in, 2 out]
        n32 = property on="P6" class="Bool (strict)"("DisabledEnum"=w90) -> ()  [unwired: 2 in, 2 out]
        n33 = property on="P8" class="Bool (strict)"("DisabledEnum"=w90) -> ()  [unwired: 2 in, 2 out]
        n34 = property on="P3" class="Bool (strict)"("DisabledEnum"=w90) -> ()  [unwired: 2 in, 2 out]
        n35 = property on="EXIT" class="Bool (strict)"("DisabledEnum"=w90) -> ()  [unwired: 2 in, 2 out]
        n36 = property on="Export" class="Bool (strict)"("DisabledEnum"=w90) -> ()  [unwired: 2 in, 2 out]
        n37 = property on="P4" class="Bool (strict)"("DisabledEnum"=w90) -> ()  [unwired: 2 in, 2 out]
        n38 = case shown="True" w92 {
          tunnel: w90 -> [_ w110]
          frame False {
          }
          frame True {
            n39 = property on="Start" class="Bool (strict)"("DisabledEnum"=w110) -> ()  [unwired: 2 in, 2 out]
          }
        }
      }
      frame "LockSwitch" {
        w114 = T2."Disabled and Grayed Out" ("無効")
        # "Set Lock Mode to the Switch"
        n40 = property on="P1" class="Bool (strict)"("DisabledEnum"=w114) -> ()  [unwired: 2 in, 2 out]
        n41 = property on="P5" class="Bool (strict)"("DisabledEnum"=w114) -> ()  [unwired: 2 in, 2 out]
        n42 = property on="P7" class="Bool (strict)"("DisabledEnum"=w114) -> ()  [unwired: 2 in, 2 out]
        n43 = property on="P2" class="Bool (strict)"("DisabledEnum"=w114) -> ()  [unwired: 2 in, 2 out]
        n44 = property on="P6" class="Bool (strict)"("DisabledEnum"=w114) -> ()  [unwired: 2 in, 2 out]
        n45 = property on="P8" class="Bool (strict)"("DisabledEnum"=w114) -> ()  [unwired: 2 in, 2 out]
        n46 = property on="P3" class="Bool (strict)"("DisabledEnum"=w114) -> ()  [unwired: 2 in, 2 out]
        n47 = property on="EXIT" class="Bool (strict)"("DisabledEnum"=w114) -> ()  [unwired: 2 in, 2 out]
        n48 = property on="Export" class="Bool (strict)"("DisabledEnum"=w114) -> ()  [unwired: 2 in, 2 out]
        n49 = property on="P4" class="Bool (strict)"("DisabledEnum"=w114) -> ()  [unwired: 2 in, 2 out]
        n50 = case shown="True" w116 {
          tunnel: w114 -> [_ w134]
          frame False {
          }
          frame True {
            n51 = property on="Start" class="Bool (strict)"("DisabledEnum"=w134) -> ()  [unwired: 2 in, 2 out]
          }
        }
      }
      frame "SetPower" {
        # "Set power of the PMT-Module"
        n52 = local read "P1"() -> (w144:bool)
        n53 = Boolean To (0,1)(Boolean=w144) -> (0, 1=w143:i16)
        n54 = To Long Integer(number=w143) -> (32bit integer=w142:i32)
        n55 = call "Set HV.vi"("HV"=w142, "handle"=w145) -> ()  [unwired: 8 in, 2 out]
      }
      frame "SetIT" {
        # "Set internal time ....."
        n56 = local read "IT"() -> (w167:i32)
        n57 = To Long Integer(number=w167) -> (32bit integer=w168:i32)
        n58 = call "Set IT.vi"("IT"=w168, "handle"=w169) -> ()  [unwired: 8 in, 2 out]
        n59 = local write "P3"(FALSE ("P3")) -> ()
      }
      frame "SetRN" {
        # "Set read number ....."
        n60 = local read "RN"() -> (w191:i32)
        n61 = To Long Integer(number=w191) -> (32bit integer=w192:i32)
        n62 = call "Set RN.vi"("RN"=w192, "handle"=w193) -> ()  [unwired: 8 in, 2 out]
        n63 = local write "P5"(FALSE ("P3")) -> ()
      }
      frame "SetStepProp" {
        # "Set Step SIze properties....."
        n64 = stacked-sequence {
          frame #0 {
            n65 = local read "WT"() -> (w230:i32)
            n66 = local read "ES"() -> (w229:i32)
            n67 = local read "SS"() -> (w231:dbl)
            n68 = local read "EP"() -> (w232:dbl)
            n69 = local read "SP"() -> (w233:dbl)
            n70 = local write "SSD"(w231) -> ()
            n71 = local write "WTD"(w230) -> ()
            n72 = local write "ESD"(w229) -> ()
            n73 = local write "SPD"(w233) -> ()
            n74 = local write "EPD"(w232) -> ()
          }
          frame #1 {
            n75 = local read "SP"() -> (w235:dbl)
            n76 = local read "EP"() -> (w236:dbl)
            n77 = local read "SS"() -> (w240:dbl)
            n78 = local read "ES"() -> (w238:i32)
            n79 = Subtract(x=w236, y=w235) -> (x-y=w234:dbl)
            n80 = Divide(x=w234, y=w240) -> (x/y=w239:dbl)
            n81 = Add(x=w239, y=w238) -> (x+y=w237:dbl)
            n82 = local write "SND"(w237) -> ()
          }
        }
        n83 = local write "P7"(FALSE) -> ()
      }
      frame "ReadPower" {
        # "Read power flag of the PMT-Module"
        n84 = local read "PowerD"() -> (w251:i32)
        n85 = call "Read HV.vi"("HV"=w251, "handle"=w250) -> ("HV out"=w249:i32)  [unwired: 7 in, 2 out]
        n86 = local write "PowerD"(w249) -> ()
        n87 = local write "P2"(FALSE ("P2")) -> ()
      }
      frame "ReadIT" {
        # "Read internal time of the PMT-Module"
        n88 = local read "ITD"() -> (w275:i32)
        n89 = call "Read IT.vi"("IT"=w275, "handle"=w274) -> ("IT out"=w273:i32)  [unwired: 7 in, 2 out]
        n90 = local write "ITD"(w273) -> ()
        n91 = local write "P4"(FALSE ("P4")) -> ()
      }
      frame "ReadRN" {
        # "Read data read number of the PMT-Module"
        n92 = local read "RND"() -> (w299:i32)
        n93 = call "Read RN.vi"("RN"=w299, "handle"=w298) -> ("RN out"=w296:i32)  [unwired: 7 in, 2 out]
        n94 = local write "RND"(w296) -> ()
        n95 = local write "P6"(FALSE ("P4")) -> ()
      }
      frame "ReadSN" {
        # "Read data sweep number of the Motorized stage"
        n96 = Increment(x=w312) -> (x+1=w313:i32)
        n97 = local write "SN"(w313) -> ()
      }
      frame "CountStart" {
        # "Conter Start!"
        n98 = local read "Correction"() -> (w341:bool)
        n99 = Boolean To (0,1)(Boolean=w341) -> (0, 1=w343:i16)
        n100 = To Long Integer(number=w343) -> (32bit integer=w342:i32)
        n101 = call "Count Start.vi"("Correction"=w342, "handle"=w344) -> ()  [unwired: 8 in, 2 out]
      }
      frame "CountStop" {
        w358 = FALSE ("Start")
        # "Add Auto Sweep button local variable here"
        # "Conter Stop!"
        n102 = local write "Auto-Sweep"(w358) -> ()
        n103 = local write "Stop"(w358) -> ()
        n104 = local write "Start"(w358) -> ()
        n105 = call "Count Stop.vi"("handle"=w369) -> ()  [unwired: 9 in, 2 out]
        n106 = Build Array (concatenate)(w367, "ActiveSwitch") -> (w366:string[])
      }
      frame "ReadData" {
        # "Read Data...."
        n107 = stacked-sequence {
          seq-local: [_ w413 _] -> [_ _ w423]
          seq-local: [_ w412 _] -> [_ _ w424]
          tunnel: w392 -> [_ w418 _]
          tunnel: w391 -> [_ _ w426]
          tunnel: [_ _ w425] -> w390
          tunnel: [_ w408 _] -> w389
          tunnel: w388 -> [_ w411 _]
          frame #0 {
            # "DB Clear!"
            n108 = Initialize Array(u32 0, 16 ("次元サイズ")) -> (w405:u32[])
            n109 = local write "DB"(w405) -> ()
          }
          frame #1 {
            n110 = local read "OLD"() -> (w415:i32)
            n111 = local read "GN"() -> (w417:i32)
            n112 = local read "DB"() -> (w416:u32[])
            n113 = call "Read Data.vi"("OLD"=w415, "DataBuf"=w416, "GateNum"=w417, "handle"=w418) -> ("OLD out"=w414:i32, "DataBuf out"=w412:u32[], "GateNum out"=w410:i32, "function return"=w413:u32)  [unwired: 3 in, 1 out]
            n114 = local write "OLD"(w414) -> ()
            n115 = local write "GN"(w410) -> ()
            n116 = local write "DB"(w412) -> ()
            n117 = Build Array(w410) -> (w409:i32[])
            n118 = Build Array (concatenate)(w411, w409) -> (w408:i32[])
          }
          frame #2 {
            # "Check Over Rang !"
            # "ADD Data DIM"
            # "Pickup Tans Data!"
            n119 = To Long Integer(number=w423) -> (32bit integer=w421:i32)
            n120 = local read "OLD"() -> (w420:i32)
            n121 = Array Subset(array=w424, length=w421) -> (w422:u32[])  [unwired: 1 in]
            n122 = Not Equal To 0?(x=w420) -> (x != 0?=w419:bool)
            n123 = local write "OVL"(w419) -> ()
            n124 = Build Array (concatenate)(w426, w422) -> (w425:u32[])
            n125 = local write "Graph"(w425) -> ()
          }
        }
      }
      frame "AutoReadData" {
        # "add reset for the graph"
        # "Read Data...."
        n126 = stacked-sequence {
          tunnel: w429 -> [w451]
          tunnel: [w450] -> w428
          tunnel: w427 -> [w449]
          frame #0 {
            n127 = Build Array (concatenate)(w449, w451) -> (w450:dbl[])
            n128 = local write "Sweep Graph"(w450) -> ()
          }
        }
      }
      frame "CountInit" {
        w460 = 0
        # "Auto"
        # "Clear Data DIM !"
        n129 = Initialize Array(w460, w460) -> (w458:i32[])
        n130 = Build Array("LockSwitch", "ReadRN", "CountStart", "ReadData", "CheckNumber") -> (w461:string[])
        n131 = Build Array (concatenate)(w467, w461) -> (w466:string[])
      }
      frame "AutoCount|nit!" {
        w493 = 0
        # "Clear Data DIM !"
        n132 = local read "SND"() -> (w480:i32)
        n133 = local read "SN"() -> (w485:i32)
        n134 = Increment(x=w480) -> (x+1=w481:i32)
        n135 = Initialize Array(w493, w493) -> (w492:i32[])
        n136 = Less?(x=w485, y=w481) -> (x < y?=w484:bool)
        n137 = case shown="True" w484 {
          tunnel: w483 -> [w509 w512]
          tunnel: [w507 w511] -> w482
          frame False {
            n138 = Build Array("AutoReadData", "AutoCheckNumber") -> (w508:string[])
            n139 = Build Array (concatenate)(w509, w508) -> (w507:string[])
          }
          frame True {
            n140 = Build Array("LockSwitch", "ReadRN", "CountStart", "ReadData", "AutoCheckNumber") -> (w518:string[])
            n141 = Build Array (concatenate)(w512, w518) -> (w511:string[])
          }
        }
      }
      frame "CheckNumber" {
        # "Add append"
        # "Add Case Strucutre outside\nsimilar to GN,"
        # "Check RN and Data lenbgth,Stop Switch ......"
        n142 = local read "Stop"() -> (w527:bool)
        n143 = local read "GN"() -> (w528:i32)
        n144 = Decrement(x=w530) -> (x-1=w529:i32)
        n145 = Less?(x=w528, y=w529) -> (x < y?=w534:bool)
        n146 = case shown="False" w534 {
          tunnel: [w549 w551] -> w531
          tunnel: w527 -> [_ w550]
          frame False {
            # "\"MotorJog\"; here"
            # "Move \"Active Swith\" to False Condition of Position Number"
            # "Add \"AutoExport Run\" here"
            n147 = local write "Start"(FALSE ("Start")) -> ()
            n148 = Build Array("CountStop", "ActiveSwitch") -> (w549:string[])
          }
          frame True {
            n149 = case shown="False" w550 {
              tunnel: [w553 w555] -> w551
              frame False {
                n150 = Build Array("ReadData", "CheckNumber") -> (w553:string[])
              }
              frame True {
                n151 = Build Array("CountStop") -> (w555:string[])
              }
            }
          }
        }
        n152 = Build Array (concatenate)(w532, w531) -> (w533:string[])
      }
      frame "AutoCheckNumber" {
        # "Add append"
        # "Add Case Strucutre outside\nsimilar to GN,"
        # "Check RN and Data lenbgth,Stop Switch ......"
        n153 = local read "Stop"() -> (w568:bool)
        n154 = local read "SND"() -> (w557:i32)
        n155 = local read "SN"() -> (w561:i32)
        n156 = Less?(x=w561, y=w557) -> (x < y?=w560:bool)
        n157 = case shown="False" w560 {
          tunnel: [w585 w595] -> w570
          tunnel: w569 -> [_ w594]
          tunnel: w568 -> [_ w591]
          tunnel: [TRUE w590] -> w563
          frame False {
            w589 = FALSE ("Start")
            n158 = local write "Auto-Sweep"(w589) -> ()
            n159 = local write "Start"(w589) -> ()
            n160 = Build Array("CountStop", "AutoExportSweep", "ActiveSwitch") -> (w585:string[])
          }
          frame True {
            n161 = local read "GN"() -> (w592:i32)
            n162 = Decrement(x=w594) -> (x-1=w593:i32)
            n163 = Less?(x=w592, y=w593) -> (x < y?=w596:bool)
            n164 = case shown="False" w596 {
              tunnel: [w598 w614] -> w595
              tunnel: w591 -> [w599 w613]
              tunnel: [w597 w612] -> w590
              frame False {
                # "\"MotorJog\"; here"
                # "Move \"Active Swith\" to False Condition of Position Number"
                # "Add \"AutoExport Run\" here"
                n165 = case shown="False" w599 {
                  tunnel: [w605 w610] -> w598
                  tunnel: [FALSE TRUE] -> w597
                  frame False {
                    n166 = Build Array("CountStop", "AutoExportRun", "AutoReadData", "ReadSN", "MotorJog", "AutoCount|nit!") -> (w605:string[])
                  }
                  frame True {
                    n167 = local write "Auto-Sweep"(TRUE) -> ()
                    n168 = Build Array("CountStop") -> (w610:string[])
                  }
                }
              }
              frame True {
                n169 = case shown="False" w613 {
                  tunnel: [w617 w621] -> w614
                  tunnel: [FALSE TRUE] -> w612
                  frame False {
                    n170 = Build Array("ReadData", "AutoCheckNumber") -> (w617:string[])
                  }
                  frame True {
                    n171 = Build Array("CountStop") -> (w621:string[])
                    n172 = local write "Auto-Sweep"(TRUE) -> ()
                  }
                }
              }
            }
          }
        }
        n173 = Build Array (concatenate)(w571, w570) -> (w572:string[])
      }
      frame "Export" {
        # "For Auto Export also add mean waveform"
        # "Get mean Data into 1D array Shift register for waveform"
        # "Gate Number is just number of count measurements"
        # "time...using array size"
        # "time...using array size"
        n174 = Array Size(array=w637) -> (size(s)=w649:i32)
        n175 = for {
          N: w649 -> [_]
          tunnel: [w664] -> w636 mode=indexing
          i -> [w666]
          n176 = local read "ITD"() -> (w668:i32)
          n177 = Add(x=1, y=w666) -> (x+y=w667:i32)
          n178 = Multiply(x=w668, y=w667) -> (x*y=w664:i32)
        }
        n179 = call <vilib>:"Std Deviation and Variance.vi"("X"=w637) -> ("mean"=w630:dbl, "standard deviation"=w629:dbl)  [unwired: 1 in, 1 out]
        n180 = Build Array(w630, w629) -> (w628:dbl[])
        n181 = Build Array(w632, w636, w637) -> (w647:u32[][])
        n182 = call-poly <vilib>:"Write Delimited Spreadsheet.vi"("1D data"=string[] ["Gate  No.", "Time [ms]", "Counts"], "append to file? (new file:F)"=FALSE, "transpose? (no:F)"=FALSE) -> ("new file path (Not A Path if cancelled)"=w646:path)  [unwired: 11 in, 1 out]
        n183 = call-poly <vilib>:"Write Delimited Spreadsheet.vi"("file path (dialog if empty)"=w646, "2D data"=w647, "append to file? (new file:F)"=TRUE, "transpose? (no:F)"=TRUE) -> ("new file path (Not A Path if cancelled)"=w642:path)  [unwired: 10 in, 1 out]
        n184 = call-poly <vilib>:"Write Delimited Spreadsheet.vi"("file path (dialog if empty)"=w642, "1D data"=string[] ["Mean", "Std. Dev."], "append to file? (new file:F)"=TRUE, "transpose? (no:F)"=FALSE) -> ("new file path (Not A Path if cancelled)"=w638:path)  [unwired: 10 in, 1 out]
        n185 = call-poly <vilib>:"Write Delimited Spreadsheet.vi"("file path (dialog if empty)"=w638, "1D data"=w628, "append to file? (new file:F)"=TRUE, "transpose? (no:F)"=FALSE) -> ()  [unwired: 10 in, 2 out]
        n186 = local write "Export"(FALSE) -> ()
      }
      frame "AutoExportRun" {
        # "For Auto Export also add mean waveform"
        # "Get mean Data into 1D array Shift register for waveform"
        # "Gate Number is just number of count measurements"
        # "time...using array size"
        # "time...using array size"
        n187 = Array Size(array=w690) -> (size(s)=w702:i32)
        n188 = for {
          N: w702 -> [_]
          tunnel: [w722] -> w689 mode=indexing
          i -> [w724]
          n189 = local read "ITD"() -> (w726:i32)
          n190 = Add(x=1, y=w724) -> (x+y=w725:i32)
          n191 = Multiply(x=w726, y=w725) -> (x*y=w722:i32)
        }
        n192 = flat-sequence {
          tunnel: w673 -> [w721]
          tunnel: [w717] -> w672
          frame #0 {
            n193 = local read "SS"() -> (w720:dbl)
            n194 = Multiply(x=w721, y=w720) -> (x*y=w718:dbl)
            n195 = local read "SP"() -> (w719:dbl)
            n196 = Add(x=w719, y=w718) -> (x+y=w717:dbl)
          }
        }
        n197 = call <vilib>:"Std Deviation and Variance.vi"("X"=w690) -> ("mean"=w679:dbl, "standard deviation"=w683:dbl)  [unwired: 1 in, 1 out]
        n198 = Build Array(w679, w683) -> (w682:dbl[])
        n199 = Number To Decimal String(number=w672) -> (decimal integer string=w671:string)  [unwired: 1 in]
        n200 = Build Array(w685, w689, w690) -> (w700:u32[][])
        n201 = Build Array (concatenate)(string[] ["Angle (deg)"], w671) -> (w669:string[])
        n202 = call-poly <vilib>:"Write Delimited Spreadsheet.vi"("file path (dialog if empty)"=w677, "1D data"=w669, "append to file? (new file:F)"=TRUE, "transpose? (no:F)"=FALSE) -> ("new file path (Not A Path if cancelled)"=w676:path)  [unwired: 10 in, 1 out]
        n203 = call-poly <vilib>:"Write Delimited Spreadsheet.vi"("file path (dialog if empty)"=w676, "1D data"=string[] ["Gate  No.", "Time [ms]", "Counts"], "append to file? (new file:F)"=TRUE, "transpose? (no:F)"=FALSE) -> ("new file path (Not A Path if cancelled)"=w699:path)  [unwired: 10 in, 1 out]
        n204 = call-poly <vilib>:"Write Delimited Spreadsheet.vi"("file path (dialog if empty)"=w699, "2D data"=w700, "append to file? (new file:F)"=TRUE, "transpose? (no:F)"=TRUE) -> ("new file path (Not A Path if cancelled)"=w695:path)  [unwired: 10 in, 1 out]
        n205 = call-poly <vilib>:"Write Delimited Spreadsheet.vi"("file path (dialog if empty)"=w695, "1D data"=string[] ["Mean", "Std. Dev."], "append to file? (new file:F)"=TRUE, "transpose? (no:F)"=FALSE) -> ("new file path (Not A Path if cancelled)"=w691:path)  [unwired: 10 in, 1 out]
        n206 = call-poly <vilib>:"Write Delimited Spreadsheet.vi"("file path (dialog if empty)"=w691, "1D data"=w682, "append to file? (new file:F)"=TRUE, "transpose? (no:F)"=FALSE) -> ("new file path (Not A Path if cancelled)"=w681:path)  [unwired: 10 in, 1 out]
        n207 = local write "Export"(FALSE) -> ()
      }
      frame "AutoExportSweep" {
        # "For Auto Export also add mean waveform"
        # "Get mean Data into 1D array Shift register for waveform"
        # "Gate Number is just number of count measurements"
        # "time...using array size"
        # "time...using array size"
        n208 = Array Size(array=w728) -> (size(s)=w753:i32)
        n209 = for {
          N: w753 -> [_]
          tunnel: [w771] -> w740 mode=indexing
          i -> [w768]
          n210 = local read "SS"() -> (w772:dbl)
          n211 = Multiply(x=w772, y=w768) -> (x*y=w769:dbl)
          n212 = local read "SP"() -> (w770:dbl)
          n213 = Add(x=w770, y=w769) -> (x+y=w771:dbl)
        }
        n214 = call <vilib>:"Std Deviation and Variance.vi"("X"=w728) -> ("mean"=w729:dbl, "standard deviation"=w734:dbl)  [unwired: 1 in, 1 out]
        n215 = Build Array(w729, w734) -> (w733:dbl[])
        n216 = Build Array(w740, w728) -> (w751:dbl[][])
        n217 = call-poly <vilib>:"Write Delimited Spreadsheet.vi"("file path (dialog if empty)"=w730, "1D data"=string[] ["Angle Itr.", "Counts Mean", ""], "append to file? (new file:F)"=TRUE, "transpose? (no:F)"=FALSE) -> ("new file path (Not A Path if cancelled)"=w750:path)  [unwired: 10 in, 1 out]
        n218 = call-poly <vilib>:"Write Delimited Spreadsheet.vi"("file path (dialog if empty)"=w750, "2D data"=w751, "append to file? (new file:F)"=TRUE, "transpose? (no:F)"=TRUE) -> ("new file path (Not A Path if cancelled)"=w746:path)  [unwired: 10 in, 1 out]
        n219 = call-poly <vilib>:"Write Delimited Spreadsheet.vi"("file path (dialog if empty)"=w746, "1D data"=string[] ["Mean", "Std. Dev."], "append to file? (new file:F)"=TRUE, "transpose? (no:F)"=FALSE) -> ("new file path (Not A Path if cancelled)"=w742:path)  [unwired: 10 in, 1 out]
        n220 = call-poly <vilib>:"Write Delimited Spreadsheet.vi"("file path (dialog if empty)"=w742, "1D data"=w733, "append to file? (new file:F)"=TRUE, "transpose? (no:F)"=FALSE) -> ("new file path (Not A Path if cancelled)"=w732:path)  [unwired: 10 in, 1 out]
        n221 = local write "Export"(FALSE) -> ()
      }
      frame "AutoSweep" {
        w775 = 0
        # "1. Create a file path (Send two strings, \"SetPosition\" and \"AutoCount|nit!\")\n2. Send to \"SetPosition\"\n2.1. Will create a Position Number Shift register\n2.2. Move stage to initial position, allow time to complete movement or add delay\n3. Send to \"AutoCount|nit!\"\n3.1. \"AutoCount|nit!\" is clone of \"Count|nit!\" but sends to \"AutoCheckNumber\", not \"CheckNumber\n3.1.1. \"AutoCheckNumber\" will check if end position, or run condition is met then send \"CountStop\" and \"ActiveSwitch\"\n3.1.2. \"AutoCheck Number\" will allow \"CountStop\" to be sent via Stop Boolean\n3.1.3. \"AutoCheckNumber\" will upon END of one run will run \"AutoExportRun\" to set file path\n3.1.3.1. \"AutoExportRun\" will add a data point to Mean Waveform after Count Stop\n3.1.4. \"AutoCheckNumber\" will upon END of sweep will run \"AutoExportSweep\" then issue \"ActiveSwitch\"\n3.1.4.1. \"AutoExportSweep\" will append final Mean Sweep waveform to file path before \"CountStop\";\"ActiveSwitch\"\n4. If End condition not met; \"MotorJog\"; \"AutoCount|nit!\"....repeats\n4.1. Will move to next position by set increment, with .net code, add delay to allow it to arrive at position"
        # "Create a File path here\nSend switch case string \"SetPosition\", which has a position number switch register"
        # "1.Position Set, create a file path\n2. Count|nit!---duplicate and create auto counter, add read sweep data for auto read\n2.0.1Checknumber end, change active switch to Auto export\n3. Auto Export ... need to make \n3.0.2Auto Export end, send to read sweep data (mean, stdev for per sweep)\n3.Export\n4.check end position, check end condition met\n5.met>end;not end >continue\n6. Jog motor\n7.repeat from 2."
        # "Create Motor Controls for setting Homing, Step size for angle, idle time(if required),"
        n222 = local write "SN"(w775) -> ()
        n223 = call-poly <vilib>:"Write Delimited Spreadsheet.vi"("append to file? (new file:F)"=FALSE) -> ("new file path (Not A Path if cancelled)"=w774:path)  [unwired: 13 in, 1 out]
        n224 = Build Array("SetPosition", "AutoCount|nit!") -> (w780:string[])
        n225 = Build Array (concatenate)(w778, w780) -> (w777:string[])
      }
      frame "MotorJog" {
        # "Move position by set increment"
        # "Add a test Jog?"
        # "Put thor labs net code here"
        n226 = stacked-sequence {
          tunnel: w804 -> [w826 w829]
          frame #0 {
            n227 = local read "SSD"() -> (w825:dbl)
            n228 = invoke class="GenericAdvancedMotorCLI" method="MoveRelative"(reference=w826, "direction"=1, "stepSize"=w825, "waitTimeout"=0) -> ()  [unwired: 2 in, 6 out]
            n229 = local read "WT"() -> (w823:i32)
            n230 = Wait (ms)(milliseconds to wait=w823) -> ()  [unwired: 1 out]
          }
          frame #1 {
            n231 = invoke class="GenericAdvancedMotorCLI" method="GetPositionCounter"(reference=w829) -> ("GetPositionCounter"=w827:i32)  [unwired: 2 in, 2 out]
            n232 = Wait (ms)(milliseconds to wait=50) -> ()  [unwired: 1 out]
            n233 = local write "PC"(w827) -> ()
          }
        }
        n234 = local write "P8"(FALSE) -> ()
      }
      frame "SetPosition" {
        n235 = stacked-sequence {
          tunnel: w834 -> [w853 w858 w861]
          frame #0 {
            n236 = local read "SPD"() -> (w852:dbl)
            n237 = invoke class="GenericAdvancedMotorCLI" method="SetMoveAbsolutePosition"(reference=w853, "position"=w852) -> ()  [unwired: 2 in, 4 out]
          }
          frame #1 {
            n238 = invoke class="GenericAdvancedMotorCLI" method="MoveAbsolute"(reference=w858, "waitTimeout"=0) -> ()  [unwired: 2 in, 4 out]
            n239 = local read "WT"() -> (w854:i32)
            n240 = Add(x=w854, y=10000) -> (x+y=w855:i32)
            n241 = Wait (ms)(milliseconds to wait=w855) -> ()  [unwired: 1 out]
          }
          frame #2 {
            n242 = invoke class="GenericAdvancedMotorCLI" method="GetPositionCounter"(reference=w861) -> ("GetPositionCounter"=w859:i32)  [unwired: 2 in, 2 out]
            n243 = Wait (ms)(milliseconds to wait=50) -> ()  [unwired: 1 out]
            n244 = local write "PC"(w859) -> ()
          }
        }
      }
      frame "", "Idle" {
        n245 = event shown="[8] \"Start\": Value Change" {
          selector: _ -> [_ _ _ _ _ _ _ _ _ _ _ _ _]
          dyn-events: _ -> [_ _ _ _ _ _ _ _ _ _ _ _ _]
          timeout: _ -> [_ _ _ _ _ _ _ _ _ _ _ _ _]
          tunnel: w873 -> [w888 w891 w894 w898 w902 w906 w910 w914 w917 w919 w922 w925 w928]
          tunnel: [w886 w890 w893 w897 w901 w905 w909 w913 w916 w918 w921 w924 w929] -> w871
          event Menu Selection (User) {
            n246 = event-data() -> ("ItemTag"=w887:string)  [unwired: 1 out]
            n247 = Build Array (concatenate)(w888, w887) -> (w886:string[])
          }
          event "EXIT": Value Change {
            n248 = event-data() -> ()  [unwired: 7 out]
            n249 = Build Array (concatenate)(w891, "Exit") -> (w890:string[])
          }
          event "P1": Value Change {
            n250 = event-data() -> ()  [unwired: 7 out]
            n251 = Build Array (concatenate)(w894, "SetPower") -> (w893:string[])
          }
          event "P2": Value Change {
            n252 = event-data() -> ()  [unwired: 7 out]
            n253 = Build Array (concatenate)(w898, "ReadPower") -> (w897:string[])
            n254 = Wait (ms)(milliseconds to wait=u32 200 ("ミリ秒待機時間")) -> ()  [unwired: 1 out]
          }
          event "P3": Value Change {
            n255 = event-data() -> ()  [unwired: 7 out]
            n256 = Build Array (concatenate)(w902, "SetIT") -> (w901:string[])
            n257 = Wait (ms)(milliseconds to wait=u32 200 ("ミリ秒待機時間")) -> ()  [unwired: 1 out]
          }
          event "P4": Value Change {
            n258 = event-data() -> ()  [unwired: 7 out]
            n259 = Build Array (concatenate)(w906, "ReadIT") -> (w905:string[])
            n260 = Wait (ms)(milliseconds to wait=u32 200 ("ミリ秒待機時間")) -> ()  [unwired: 1 out]
          }
          event "P5": Value Change {
            n261 = event-data() -> ()  [unwired: 7 out]
            n262 = Build Array (concatenate)(w910, "SetRN") -> (w909:string[])
            n263 = Wait (ms)(milliseconds to wait=u32 200 ("ミリ秒待機時間")) -> ()  [unwired: 1 out]
          }
          event "P6": Value Change {
            n264 = event-data() -> ()  [unwired: 7 out]
            n265 = Build Array (concatenate)(w914, "ReadRN") -> (w913:string[])
            n266 = Wait (ms)(milliseconds to wait=u32 200 ("ミリ秒待機時間")) -> ()  [unwired: 1 out]
          }
          event "Start": Value Change {
            n267 = event-data() -> ()  [unwired: 7 out]
            n268 = Build Array (concatenate)(w917, "CountInit") -> (w916:string[])
          }
          event "Export": Value Change {
            n269 = event-data() -> ()  [unwired: 7 out]
            n270 = Build Array (concatenate)(w919, "Export") -> (w918:string[])
          }
          event "P7": Value Change {
            n271 = event-data() -> ()  [unwired: 7 out]
            n272 = Build Array (concatenate)(w922, "SetStepProp") -> (w921:string[])
          }
          event "P8": Value Change {
            n273 = event-data() -> ()  [unwired: 7 out]
            n274 = Build Array (concatenate)(w925, "MotorJog") -> (w924:string[])
          }
          event "Auto-Sweep": Value Change {
            n275 = event-data() -> ()  [unwired: 7 out]
            n276 = Build Array (concatenate)(w928, "AutoSweep") -> (w929:string[])
            n277 = Wait (ms)(milliseconds to wait=200) -> ()  [unwired: 1 out]
          }
        }
        n278 = Build Array (concatenate)("", w871) -> (w870:string[])
      }
      frame "Error", Default {
        n279 = Concatenate Strings("Error  Case Name .....", "\r\n", w938) -> (w940:string)
        n280 = One Button Dialog(message=w940) -> (true=w939:bool)  [unwired: 1 out]
        n281 = stacked-sequence {
          tunnel: w939 -> [_]
          frame #0 {
            n282 = Stop() -> ()  [unwired: 1 out]
          }
        }
      }
      frame "Exit" {
        # "See you again ......"
        n283 = call "Close.vi"("Handle"=w964) -> ()  [unwired: 9 in, 2 out]
      }
    }
    n284 = local write "PC"(w17) -> ()
    n285 = call "SM_CaseErase.vi"("Input"=w41) -> ("Output"=w40:string[])  [unwired: 10 out]
  }
  n286 = invoke class="BenchtopStepperControl" method="CloseDevice"(reference=w10) -> ()  [unwired: 2 in, 3 out]
